vi "main OP500P.vi"() -> ()   [LabVIEW 2020]
uses:
  SubVI/Contactor_Status.ctl
  SubVI/OP500Z8_state_P.ctl
  <userlib>/PCAN Basic/Controls/BaudrateEenum.ctl
  <userlib>/PCAN Basic/Controls/Channel.ctl
  ZEN8 Semi Auto EMC/OP700/SubVI/FGV/FGV_Enum.ctl
  C:/Users/elhajj/OneDrive - FORSEE POWER/Bureau/Support banc de test/Ligne ZENPLUS/Code LabVIEW/CODE/02 SLIM ZEN WS 500/SubVi/FGV.ctl
  13eb9333-f902-445b-951f-98894687dcd3.vi
  af390806-a127-4432-953e-00834710d83e.vi
  5474c4f2-57a2-4d07-9e76-894820534c83.vi
  c213c121-1213-470d-a8c3-6a59dea4dab1.vi
  060584ca-cb65-487f-8f54-703ff4f80a18.vi
  4a804ed1-565a-41e0-a699-ae70de0a1211.vi
  bf7a2284-f80f-49aa-8a3b-6e4a3f45e645.vi
  VG/VG_Barre_Progression_ISO_P.vi
  VG/VG_Ibms.vi
  VG/VG_progressBar_P.vi
  DiagTool/RAMPAGE V1.0/VI/CheminDeBase.vi
  VG/VG_DCIR+OUIouNON_P.vi
  <vilib>/Utility/file.llb/Read Delimited Spreadsheet (string).vi
  VG/VG_Conti.vi
  VG/VG_ISOmin_P.vi
  VG/VG_OCV70min_P.vi
  VG/VG_OCV70max_P.vi
  VG/VG_OCV30max_P.vi
  VG/VG_OCV30min_P.vi
  VG/IS30%_P.vi
  VG/VG_DCIRmax_P.vi
  VG/VG_DCIRmin_P.vi
  <userlib>/PCAN Basic/PCANBasic.lvlib
  <userlib>/Alex_Peak_lib/PEAK_lib_ALEX.lvlib
panel:
  out "Courant BMS (A)":dbl
  out "Consigne ITECH (A)":dbl
  out "Contacteur Status":T1
  out "Boolean":bool
  out "DCIR+ ?":bool
  out "Barre de progression ISO":dbl(slide) scale=0.0..100.0
  out "VISA OUT":T2
  out "IS30% ?":bool
  out "Cluster":T3
  out "progression":dbl(slide) scale=0.0..100.0
  out "errout":errorcluster caption="sortie d'erreur"
  out "STOP":bool
  out "TOP":string
  out "DRAW":picture
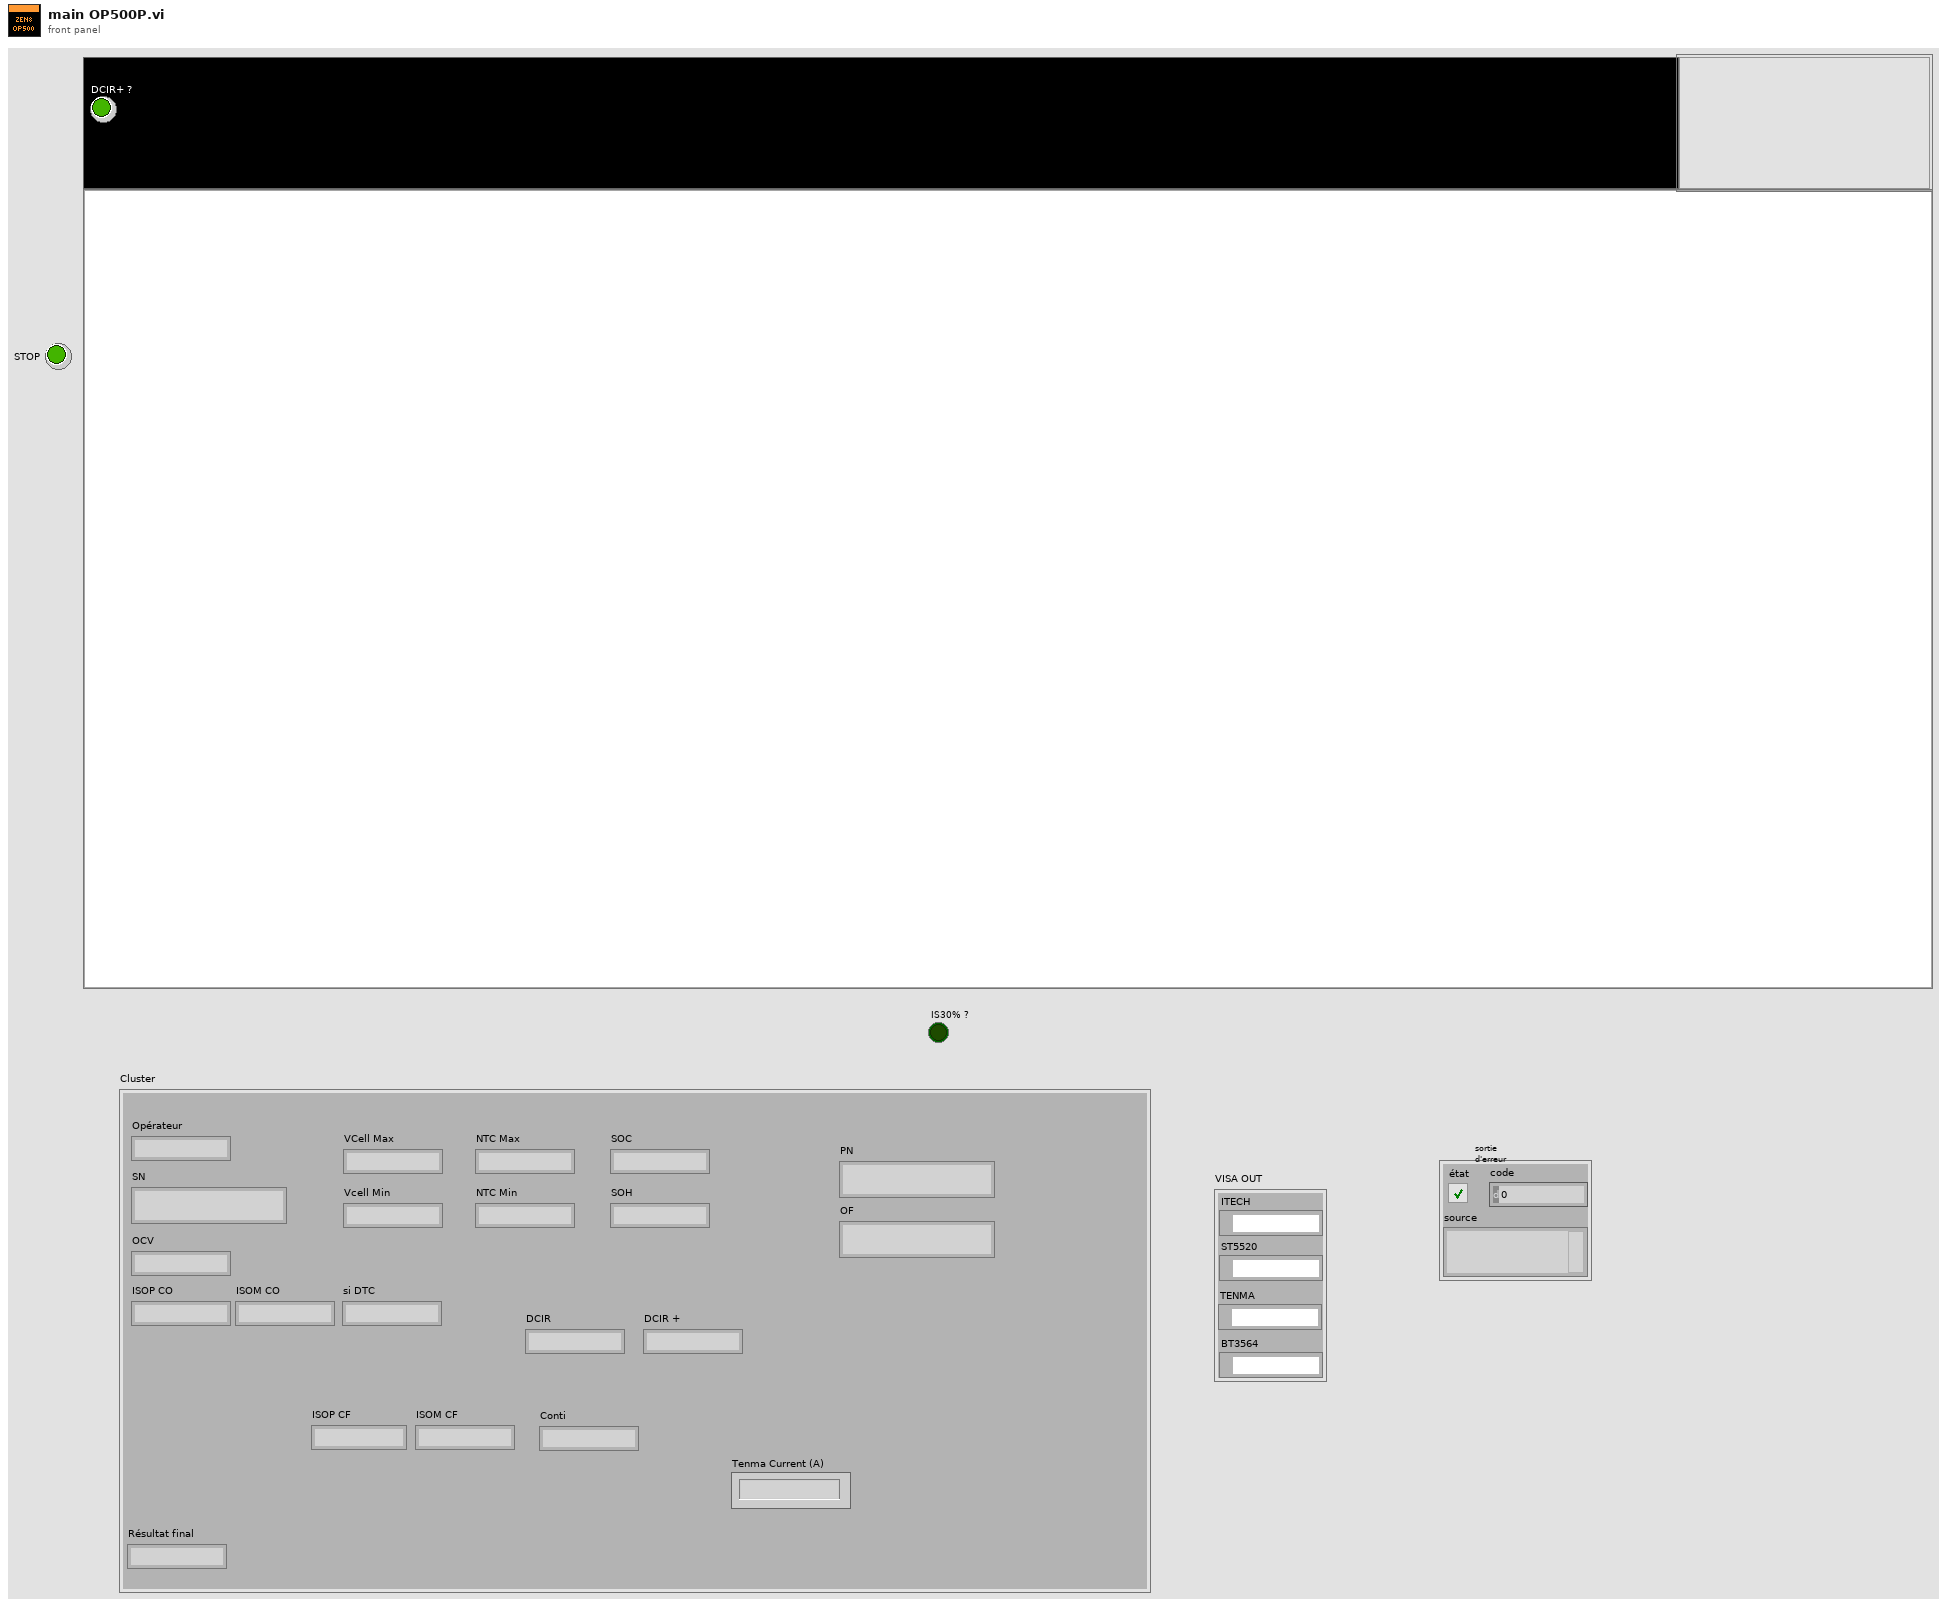
[diagram p1: front panel]
types:
  T1 = typedef "Contactor_Status.ctl" = bool
  T2 = cluster{"ITECH":refnum<visa-resource-name>, "ST5520":refnum<visa-resource-name>, "TENMA":refnum<visa-resource-name>, "BT3564":refnum<visa-resource-name>}
  T3 = cluster{"Opérateur":string, "OCV":string, "ISOP CO":string, "ISOM CO":string, "Résultat final":string, "SN":string, "DCIR":string, "si DTC":string, "Vcell Min":string, "VCell Max":string, "NTC Max":string, "NTC Min":string, "SOC":string, "SOH":string, "PN":string, "OF":string, "DCIR +":string, "Conti":string, "ISOP CF":string, "ISOM CF":string, "Tenma Current (A)":string}
  T4 = typedef "PCANBasic.lvlib/Channel.ctl" = enum16{"PCAN_NONEBUS", "not used1", "not used2", "not used3", "not used4", "not used5", "not used6", "not used7", "not used8", "not used9", "not used10", "not used11", "not used12", "not used13", "not used14", "not used15", "not used16", "not used17", "not used18", "not used19", "not used20", "not used21", "not used22", "not used23", "not used24", "not used25", "not used26", "not used27", "not used28", "not used29", "not used30", "not used31", "not used32", "PCAN_ISABUS1", "PCAN_ISABUS2", "PCAN_ISABUS3", "PCAN_ISABUS4", "PCAN_ISABUS5", "PCAN_ISABUS6", "PCAN_ISABUS7", "PCAN_ISABUS8", "not used41", "not used42", "not used43", "not used44", "not used45", "not used46", "not used47", "not used48", "PCAN_DNGBUS1", "not used50", "not used51", "not used52", "not used53", "not used54", "not used55", "not used56", "not used57", "not used58", "not used59", "not used60", "not used61", "not used62", "not used63", "not used64", "PCAN_PCIBUS1", "PCAN_PCIBUS2", "PCAN_PCIBUS3", "PCAN_PCIBUS4", "PCAN_PCIBUS5", "PCAN_PCIBUS6", "PCAN_PCIBUS7", "PCAN_PCIBUS8", "not used73", "not used74", "not used75", "not used76", "not used77", "not used78", "not used79", "not used80", "PCAN_USBBUS1", "PCAN_USBBUS2", "PCAN_USBBUS3", "PCAN_USBBUS4", "PCAN_USBBUS5", "PCAN_USBBUS6", "PCAN_USBBUS7", "PCAN_USBBUS8", "Not used89", "Not used90", "Not used91", "Not used92", "Not used93", "Not used94", "Not used95", "Not used96", "PCAN_PCCBUS1", "PCAN_PCCBUS2"}
  T5 = typedef "PCANBasic.lvlib/BaudrateEenum.ctl" = enum16{"CAN_Baud_1M", "CAN_Baud_800K", "CAN_BAUD_500K", "CAN_BAUD_250K", "CAN_BAUD_125K", "CAN_BAUD_100K", "CAN_BAUD_95K", "CAN_BAUD_83K", "CAN_BAUD_50K", "CAN_BAUD_47K", "CAN_BAUD_33K", "CAN_BAUD_20K", "CAN_BAUD_10K", "CAN_BAUD_5K", "User Baudrate"}
  T6 = typedef "FGV_Enum.ctl" = enum16{"GET", "SET"}
  T7 = typedef "OP500Z8_state_P.ctl" = enum16{"BuildSys", "Soft", "FinVol", "Null", "Demarrage", "Init", "Scan", "Montage", "Conti", "Iso", "CANCOM", "OCV", "CurrentTest", "GoDCIR", "DataDyn", "Demontage", "Crash", "Next", "DCIR", "EXIT", "LogErr", "DTC"}
  T8 = typedef "FGV.ctl" = enum16{"GET", "SET", "RAZ"}
  T9 = cluster{"OCV":string, "Current":string, "VCell Max":string, "VCell Min":string, "NTC Max":string, "NTC Min":string, "SOC":string, "SOH":string, "DTC":string, "DCIR -":string, "DCIR +":string}
  T10 = cluster{"Opérateur":string, "OCV":string, "ISOP":string, "ISOM":string, "Résultat final":string, "SN":string, "DCIR":string, "si DTC":string, "Vcell Min":string, "VCell Max":string, "NTC Max":string, "NTC Min":string, "SOC":string, "SOH":string, "PN":string, "OF":string, "DCIR+":string, "Conti":string, "ISOP CF":string, "ISOM CF":string, "Tenma Current (A)":string}
  T11 = typedef "imagedata.ctl" = cluster{"image type":i32, "image depth":i32, "image":u8[], "mask":u8[], "colors":u32[], "Rectangle":cluster{"left":i16, "top":i16, "right":i16, "bottom":i16}}
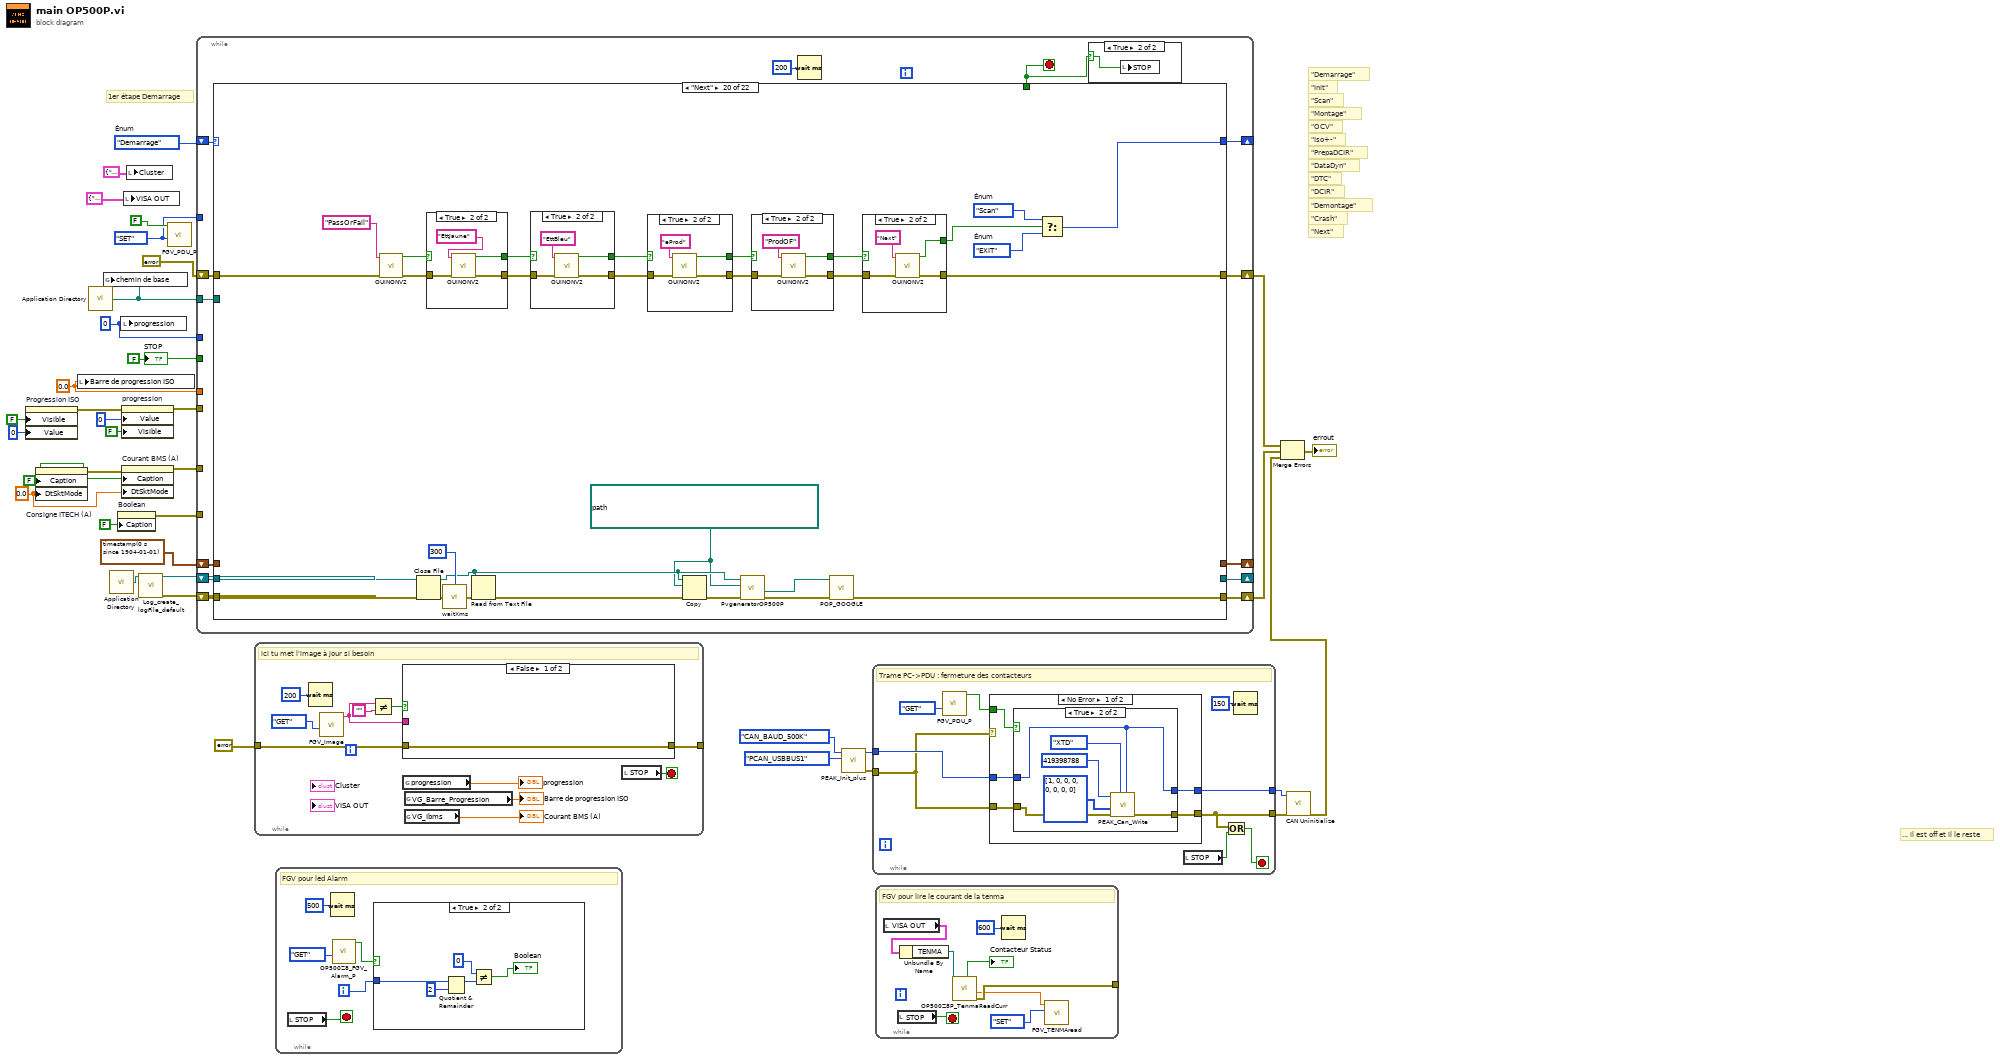
[diagram p0: block diagram]
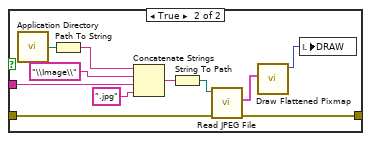
[diagram p5: hidden frame]
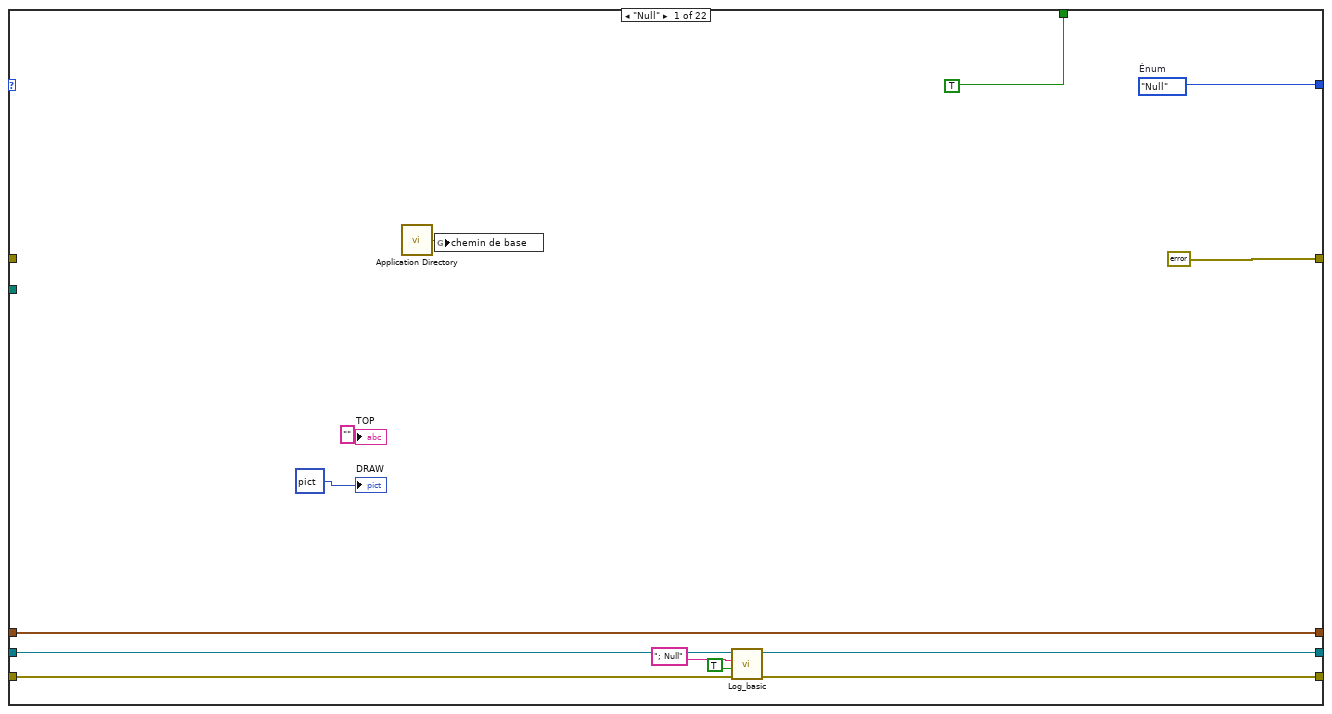
[diagram p7: hidden frame]
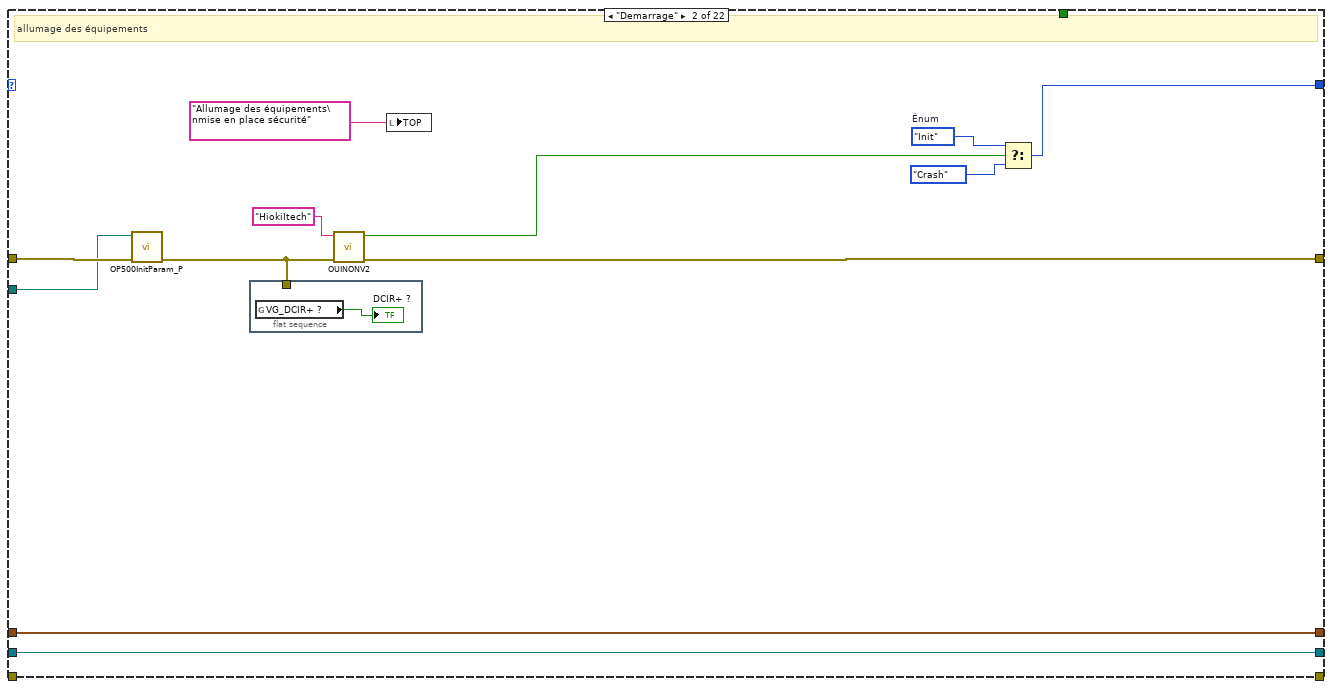
[diagram p8: hidden frame]
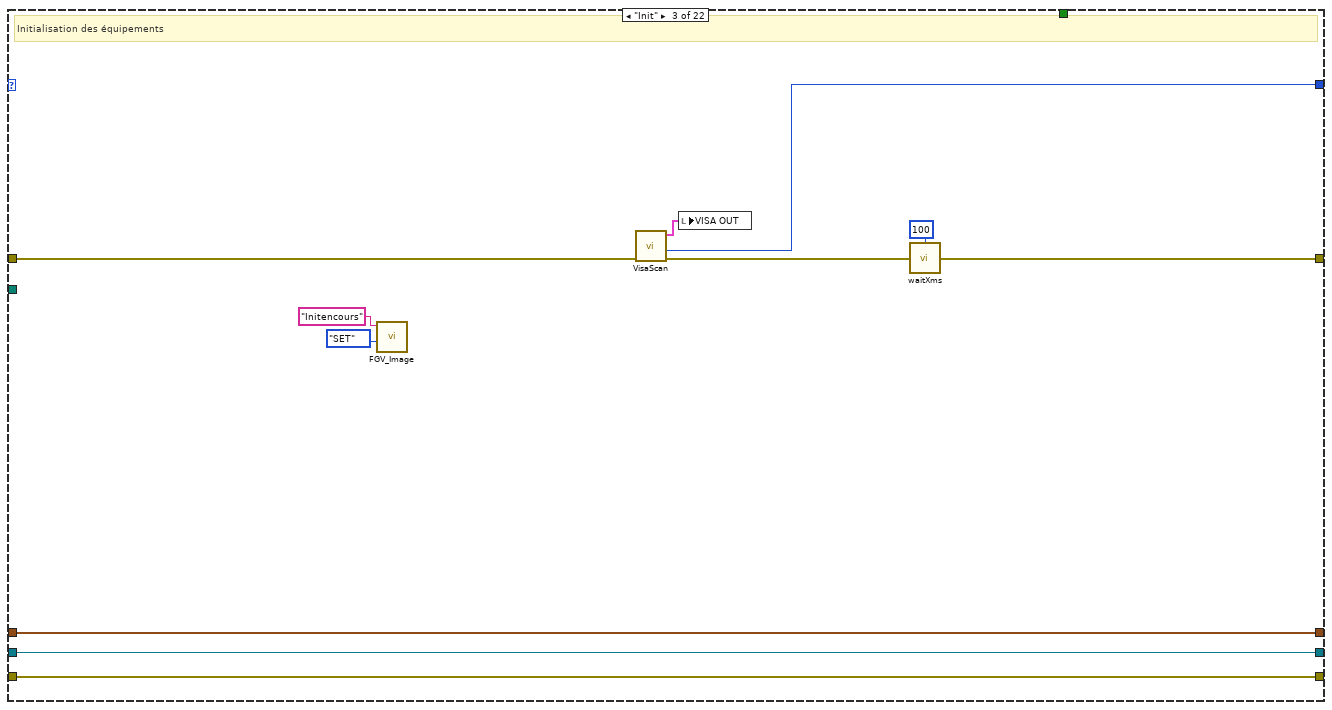
[diagram p9: hidden frame]
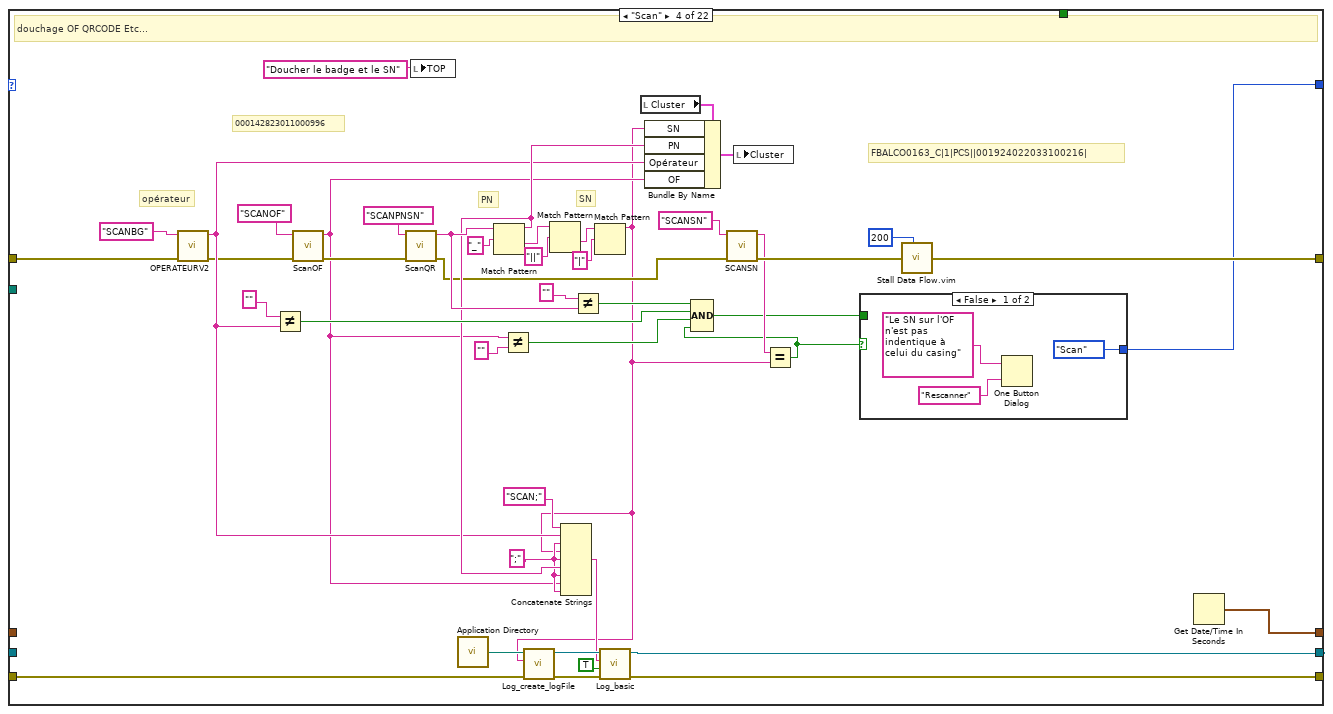
[diagram p10: hidden frame]
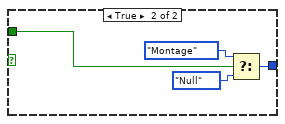
[diagram p11: hidden frame]
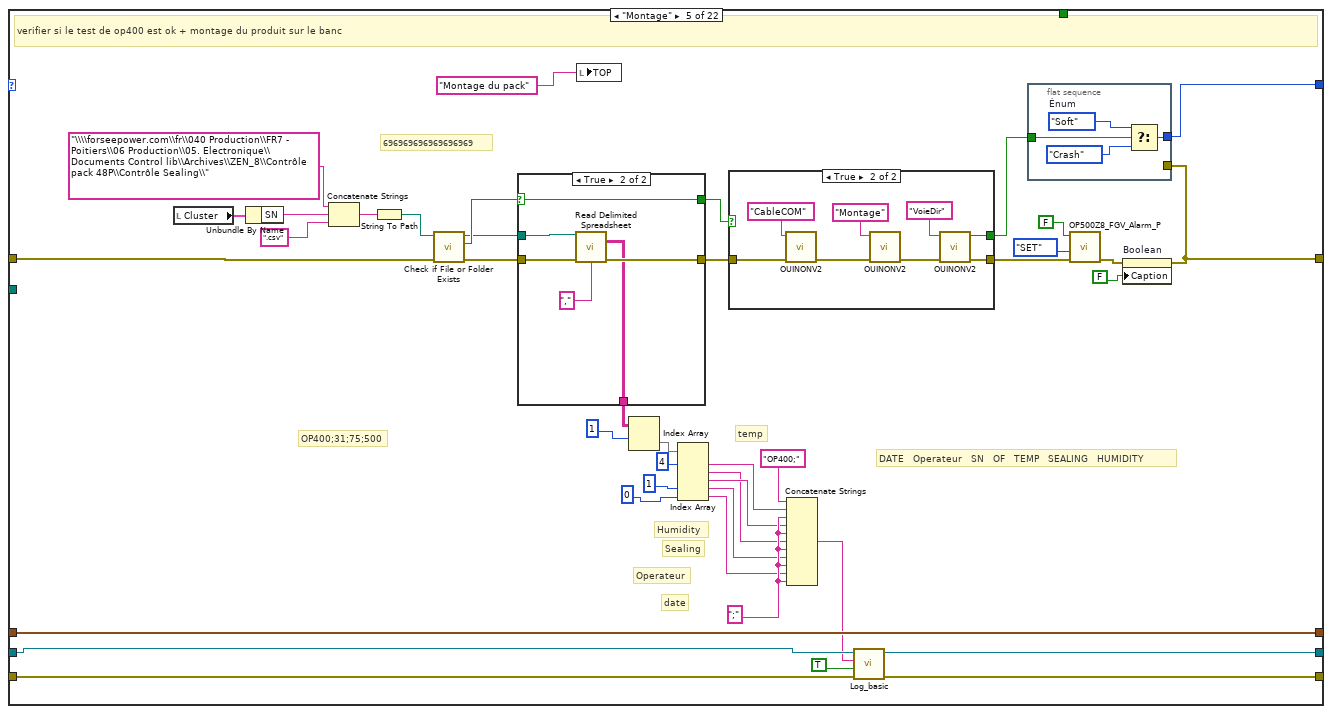
[diagram p12: hidden frame]
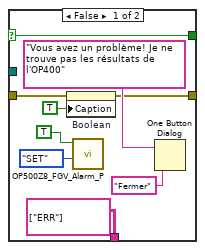
[diagram p14: hidden frame]
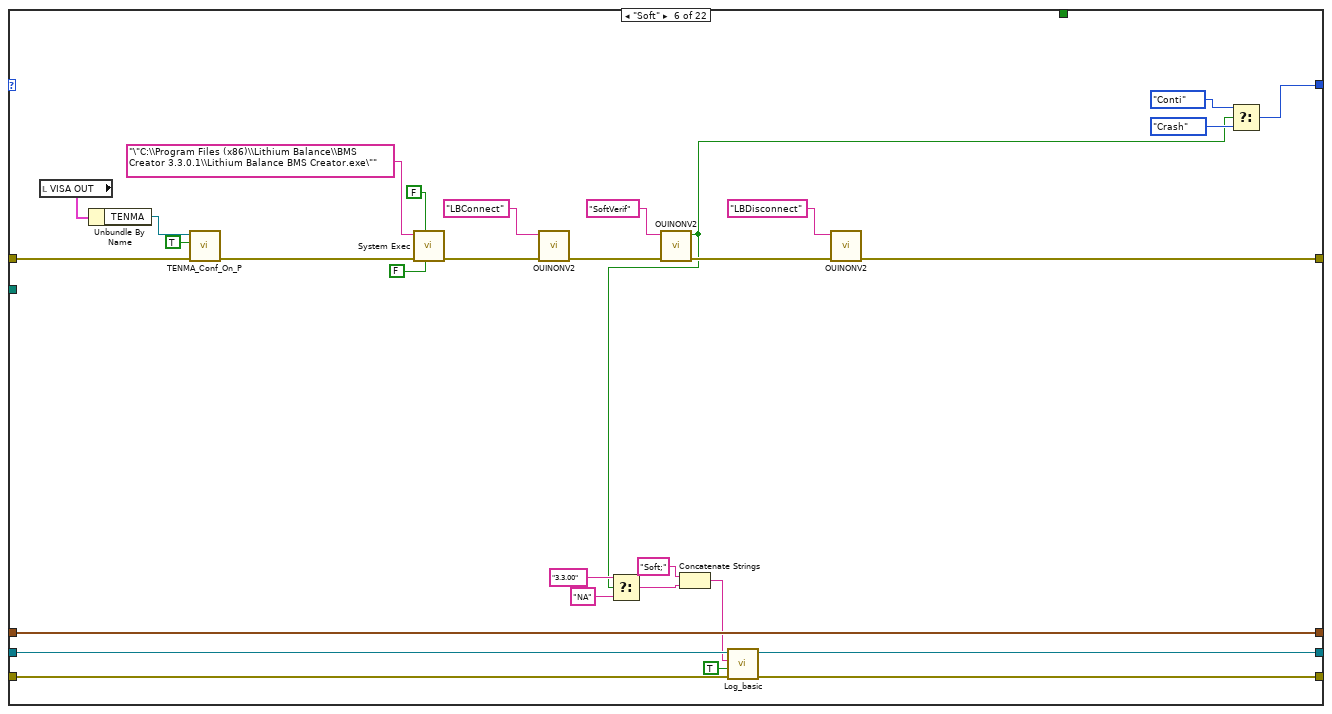
[diagram p15: hidden frame]
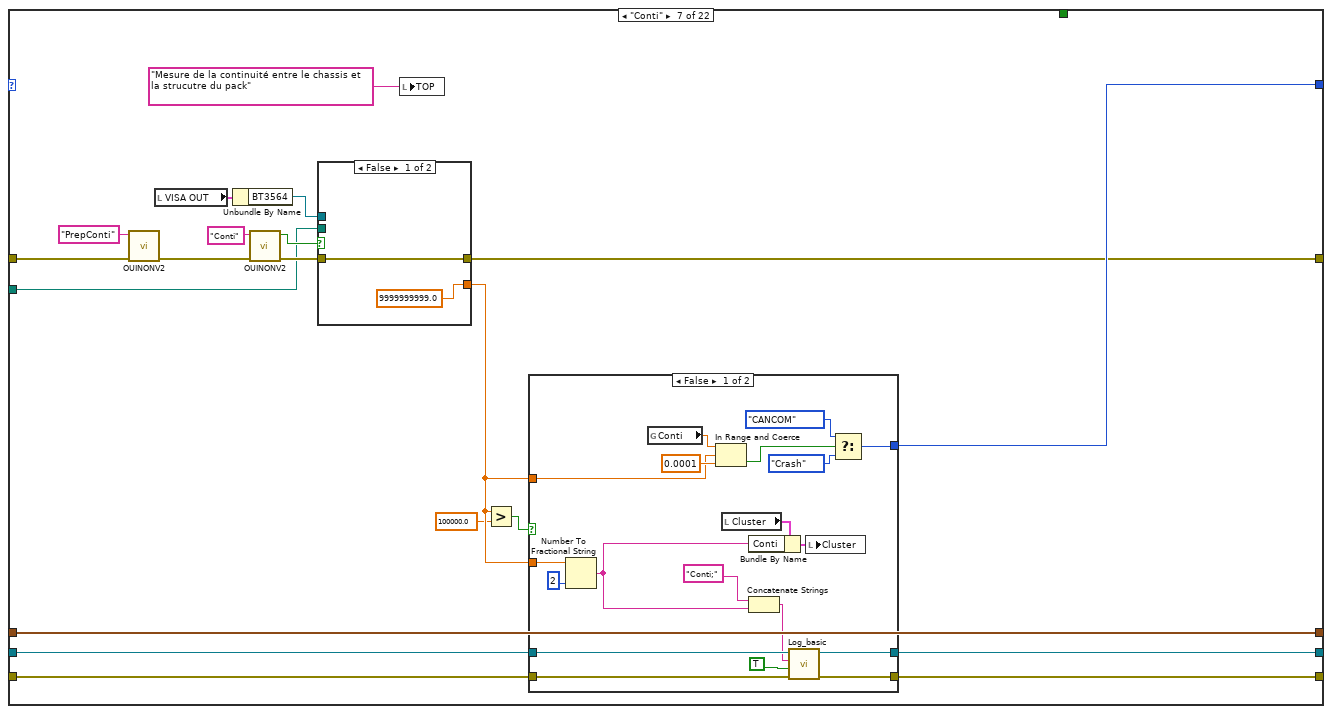
[diagram p16: hidden frame]
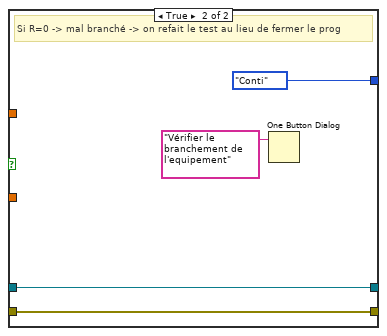
[diagram p17: hidden frame]
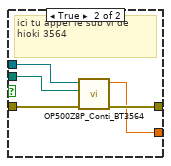
[diagram p18: hidden frame]
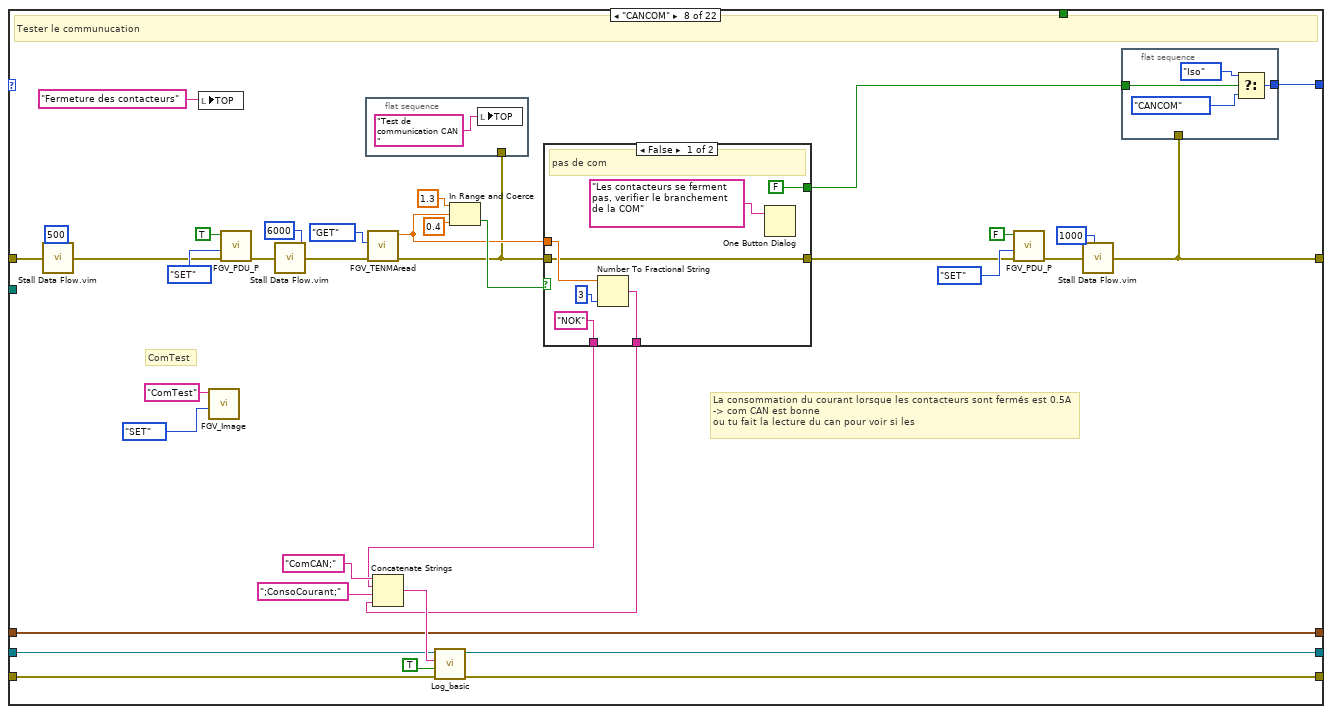
[diagram p19: hidden frame]
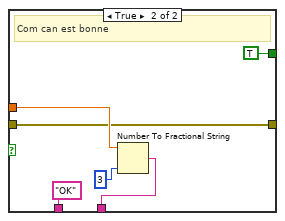
[diagram p20: hidden frame]
diagram:
  w7 = 0.0 ("Consigne ITECH (A)")
  w10 = FALSE ("Caption")
  w16 = FGV_Enum."SET" ("Énum")
  w18 = 0.0 ("Barre de progression ISO")
  w27 = u8 0 ("progression")
  w22 = OP500Z8_state_P."Demarrage"  # Énum
  w33 = FALSE ("STOP")
  # "\"Next\""
  # "\"DCIR\""
  # "\"DTC\""
  # "1er étape Demarrage"
  # "\"Crash\""
  # "\"Demontage\""
  # "\"DataDyn\""
  # "\"Iso+-\""
  # "\"Montage\""
  # "\"Scan\""
  # "\"Init\""
  # "\"Demarrage\""
  # "\"OCV\""
  # "\"PrepaDCIR\""
  # "... il est off et il le reste"
  n1 = property on="Progression ISO" class="Slide (strict)"("Visible"=FALSE, "Value"=u8 0 ("Glissière")) -> (error out=w11:errorcluster)  [unwired: 2 in, 1 out]
  n2 = property on="Consigne ITECH (A)" class="DigNum (strict)"("Caption"=w10, "DtSktMode"=w7) -> (error out=w8:errorcluster)  [unwired: 2 in, 1 out]
  n3 = local write "Barre de progression ISO"(w18) -> ()
  n4 = call <vilib>:"Application Directory.vi"() -> ("Application Directory"=w32:path)
  n5 = global write "CheminDeBase.vi" "chemin de base"(w32) -> ()
  n6 = call <vilib>:"Application Directory.vi"() -> ("Application Directory"=w30:path)
  n7 = property on="Boolean" class="Bool (strict)"("Caption"=FALSE) -> (error out=w13:errorcluster)  [unwired: 2 in, 1 out]
  n8 = local write "progression"(w27) -> ()
  n9 = property on="progression" class="Slide (strict)"(error in=w11, "Value"=u8 0 ("progression"), "Visible"=FALSE) -> (error out=w25:errorcluster)  [unwired: 1 in, 1 out]
  n10 = property on="Courant BMS (A)" class="DigNum (strict)"(error in=w8, "Caption"=w10, "DtSktMode"=w7) -> (error out=w9:errorcluster)  [unwired: 1 in, 1 out]
  n11 = local write "VISA OUT"(T2 {"ITECH"="", "ST5520"="", "TENMA"="", "BT3564"=""} ("VISA OUT")) -> ()
  n12 = local write "Cluster"(T3 {"Opérateur"="", "OCV"="", "ISOP CO"="", "ISOM CO"="", "Résultat final"="", "SN"="", "DCIR"="", "si DTC"="", "Vcell Min"="", "VCell Max"="", "NTC Max"="", "NTC Min"="", "SOC"="", "SOH"="", "PN"="", "OF"="", "DCIR +"="", "Conti"="", "ISOP CF"="", "ISOM CF"="", "Tenma Current (A)"=""} ("Cluster")) -> ()
  n13 = call <userlib>:"Log_create_logFile_default.vi"("appdir"=w30) -> ("errout"=w31:errorcluster, "Fichier à flux d'octets en sortie"=w34:refnum<file>)  [unwired: 9 in]
  n14 = call "FGV_PDU_P.vi"("Énum"=w16, "IN"=FALSE) -> ()  [unwired: 8 in, 2 out]
  n15 = while {
    shift-right: [w49] -> w36
    shift-left: errorcluster {"status"=FALSE, "code"=0, "source"=""} ("error out") -> [w40]
    shift-right: [w45] -> w35
    shift-left: w31 -> [w48]
    shift-right: [w46] -> _
    shift-left: w34 -> [w47]
    tunnel: w32 -> [w43]
    tunnel: w33 -> [_]
    shift-right: [w41] -> _
    shift-left: timestamp(0 s since 1904-01-01) ("seconds since 1Jan1904") -> [w42]
    tunnel: w27 -> [_]
    tunnel: w25 -> [_]
    shift-right: [w38] -> _
    shift-left: w22 -> [w39]
    tunnel: w18 -> [_]
    tunnel: w16 -> [_]
    tunnel: w13 -> [_]
    tunnel: w9 -> [_]
    stop <- w44 stop-if-true
    n16 = case "Structure Condition" shown="\"Next\"" w39 {
      tunnel: w40 -> [_ w69 w83 w133 w170 w214 w244 w292 w350 w463 w524 w607 w727 w750 w776 w796 w837 w854 w862 w898 w951 w957]
      tunnel: [errorcluster {"status"=FALSE, "code"=0, "source"=""} ("errin") w67 w79 w99 w151 w232 w241 w297 w359 w470 w529 w600 w721 w749 w775 w801 w837 w848 w863 w887 w950 w958] -> w49
      tunnel: w48 -> [w60 _ w88 w129 w160 w228 w258 w324 w396 w486 w588 w608 w736 w758 w783 w817 w842 w856 w882 w914 _ _]
      tunnel: w47 -> [w61 w76 w87 _ w158 w227 w260 w323 w395 w488 w590 w609 w734 w757 w788 w819 w844 w857 w883 w915 _ _]
      tunnel: [w58 w76 w87 w131 w141 w226 w256 w317 w394 w484 w586 w609 w733 w756 w789 w820 w845 w857 _ _ _ _] -> w46
      tunnel: [w59 _ w88 w132 w159 w229 w257 w318 w397 w485 w587 w608 w735 w758 w790 w821 w846 w856 w872 w903 _ _] -> w45
      tunnel: [TRUE _ _ _ _ _ _ _ _ _ _ _ _ _ _ _ _ FALSE w884 _ _ _] -> w44
      tunnel: w43 -> [_ w65 _ _ _ _ w249 _ w373 _ _ _ _ _ _ _ _ _ _ _ _ _]
      tunnel: w42 -> [w54 w75 w86 _ w181 w240 w259 w322 w393 w487 w589 w611 w726 _ _ _ _ w853 _ _ _ _]
      tunnel: [w54 w75 w86 w120 w181 w240 w259 w322 w393 w487 w589 w611 w726 _ _ _ _ w853 _ _ _ _] -> w41
      tunnel: [w52 w70 w82 w90 w178 w218 w248 w320 w386 w469 w556 w606 w715 w746 w778 w814 w839 w849 w867 w904 w947 w959] -> w38
      frame "Null" {
        w52 = OP500Z8_state_P."Null"  # Énum
        n17 = call <vilib>:"Application Directory.vi"() -> ("Application Directory"=w64:path)
        n18 = global write "CheminDeBase.vi" "chemin de base"(w64) -> ()
        n19 = call <userlib>:"Log_basic.vi"("errin"=w60, "date?"=TRUE, "chaîne"="; Null", "in"=w61) -> ("sortie d'erreur"=w59:errorcluster, "refnum en sortie"=w58:refnum<file>)  [unwired: 6 in]
        "DRAW" <- picture data[5B] ("DRAW")
        "TOP" <- "" ("TOP")
      }
      frame "Demarrage" {
        w72 = OP500Z8_state_P."Init"  # Énum
        # "allumage des équipements"
        n20 = call "OP500InitParam_P.vi"("errin"=w69, "pathin"=w65) -> ("errout"=w66:errorcluster)  [unwired: 9 in]
        n21 = flat-sequence {
          tunnel: w66 -> [_]
          frame #0 {
            n22 = global read "VG_DCIR+OUIouNON_P.vi" "VG_DCIR+ ?"() -> (→"DCIR+ ?":bool)
          }
        }
        n23 = call <userlib>:"OUINONV2.vi"("errin"=w66, "image"="HiokiItech") -> ("error out"=w67:errorcluster, "Booléen"=w68:bool)  [unwired: 8 in]
        n24 = local write "TOP"("Allumage des équipements\nmise en place sécurité" ("TOP")) -> ()
        n25 = Select ("Sélectionner")(t=w72, s=w68, f=OP500Z8_state_P."Crash" ("cas faux")) -> (s? t:f=w70:T7)
      }
      frame "Init" {
        # "Initialisation des équipements"
        n26 = call "FGV_Image.vi"("Énum"=FGV."SET", "IN"="Initencours") -> ()  [unwired: 9 in, 1 out]
        n27 = call <userlib>:"VisaScan.vi"("errin"=w83) -> ("errout"=w80:errorcluster, "NextStep"=w82:T7, "VISA OUT"=w78:T2)  [unwired: 8 in]
        n28 = local write "VISA OUT"(w78) -> ()
        n29 = call <userlib>:"waitXms.vi"("attente (ms)"=u32 100, "errin"=w80) -> ("errout"=w79:errorcluster)  [unwired: 13 in]
      }
      frame "Scan" {
        w103 = ";" ("chaîne")
        # "SN"
        # "PN"
        # "FBALCO0163_C|1|PCS||001924022033100216|"
        # "000142823011000996"
        # "opérateur"
        # "douchage OF QRCODE Etc..."
        n30 = call "OPERATEURV2.vi"("errin"=w133, "IN"="SCANBG") -> ("error out"=w102:errorcluster, "Dataout"=w107:string)  [unwired: 8 in]
        n31 = Not Equal?(x="", y=w107) -> (x != y?=w121:bool)
        n32 = call <userlib>:"ScanOF.vi"("errin"=w102, "image"="SCANOF") -> ("error out"=w101:errorcluster, "OF"=w97:string)  [unwired: 8 in]
        n33 = call <userlib>:"ScanQR.vi"("errin"=w101, "image"="SCANPNSN") -> ("error out"=w96:errorcluster, "OF"=w114:string)  [unwired: 7 in, 1 out]
        n34 = local write "TOP"("Doucher le badge et le SN" ("TOP")) -> ()
        n35 = call <vilib>:"Application Directory.vi"() -> ("Application Directory"=w130:path)
        n36 = Match Pattern(string=w114, regular expression="_" ("expression régulière")) -> (before substring=w108:string, after substring=w112:string)  [unwired: 1 in, 2 out]
        n37 = Not Equal?(x=w97, y="") -> (x != y?=w104:bool)
        n38 = Match Pattern(string=w112, regular expression="||" ("expression régulière")) -> (after substring=w110:string)  [unwired: 1 in, 3 out]
        n39 = Not Equal?(x="", y=w114) -> (x != y?=w122:bool)
        n40 = Match Pattern(string=w110, regular expression="|" ("expression régulière")) -> (before substring=w92:string)  [unwired: 1 in, 3 out]
        n41 = call <userlib>:"Log_create_logFile.vi"("errin"=w129, "toute l'expression"=w92, "Application Directory"=w130) -> ("sortie d'erreur"=w127:errorcluster, "Fichier à flux d'octets en sortie"=w128:refnum<file>)  [unwired: 7 in]
        n42 = Concatenate Strings("SCAN;" ("chaîne"), w107, w103, w92, w103, w108, w103, w97, w103) -> (w125:string)
        n43 = call <userlib>:"Log_basic.vi"("errin"=w127, "date?"=TRUE, "chaîne"=w125, "in"=w128) -> ("sortie d'erreur"=w132:errorcluster, "refnum en sortie"=w131:refnum<file>)  [unwired: 6 in]
        n44 = local read "Cluster"() -> (w116:T3)
        n45 = Bundle By Name(cluster=w116, "SN"=w92, "PN"=w108, "Opérateur"=w107, "OF"=w97) -> (w115:T3)
        n46 = call <userlib>:"SCANSN.vi"("errin"=w96, "image"="SCANSN") -> ("error out"=w95:errorcluster, "SN"=w93:string)  [unwired: 8 in]
        n47 = local write "Cluster"(w115) -> ()
        n48 = Equal?(x=w93, y=w92) -> (x = y?=w91:bool)
        n49 = Compound Arithmetic op=AND ("Opérateur arithmétique")(w122, w121, w104, w91) -> (w89:bool)
        n50 = case shown="False" w91 {
          tunnel: [OP500Z8_state_P."Scan" ("cas faux") w138] -> w90
          tunnel: w89 -> [_ w137]
          frame False {
            n51 = One Button Dialog(message="Le SN sur l'OF n'est pas indentique à celui du casing", button name ("OK")="Rescanner" ("nom du bouton (\"OK\")")) -> ()  [unwired: 1 out]
          }
          frame True {
            n52 = Select ("Sélectionner")(t=OP500Z8_state_P."Montage" ("Énum"), s=w137, f=OP500Z8_state_P."Null" ("cas faux")) -> (s? t:f=w138:T7)
          }
        }
        n53 = call "Stall Data Flow.vim"("value in"=w95, "milliseconds to wait"=u32 200) -> ("value out"=w99:errorcluster)  [unwired: 1 out]
        n54 = Get Date/Time In Seconds() -> (seconds since 1Jan1904=w120:timestamp)
      }
      frame "Montage" {
        w150 = ";" ("string")
        # "date"
        # "OP400;31;75;500"
        # "Sealing"
        # "Operateur"
        # "Humidity"
        # "temp"
        # "DATE   Operateur   SN   OF   TEMP   SEALING   HUMIDITY"
        # "696969696969696969"
        # "verifier si le test de op400 est ok + montage du produit sur le banc"
        n55 = local read "Cluster"() -> (w177:T3)
        n56 = Unbundle By Name(w177) -> ("SN"=w176:string)
        n57 = Concatenate Strings("\\\\forseepower.com\\fr\\040 Production\\FR7 - Poitiers\\06 Production\\05. Electronique\\Documents Control lib\\Archives\\ZEN_8\\Contrôle pack 48P\\Contrôle Sealing\\" ("string"), w176, ".csv" ("string")) -> (w173:string)
        n58 = String To Path(string=w173) -> (path=w171:path)
        n59 = call <vilib>:"Check if File or Folder Exists.vi"("error in (no error)"=w170, "path"=w171) -> ("error out"=w169:errorcluster, "file or folder exists?"=w168:bool, "dup path"=w166:path)  [unwired: 7 in]
        n60 = case shown="True" w168 {
          selector: w168 -> [w204 w207]
          tunnel: [w199 w209] -> w172
          tunnel: w169 -> [w200 w208]
          tunnel: [w204 w207] -> w167
          tunnel: w166 -> [_ w206]
          tunnel: [string[][] [["ERR"]] ("all rows") w205] -> w153
          frame False {
            n61 = property on="Boolean" class="Bool (strict)"(error in=w200, "Caption"=TRUE) -> (error out=w199:errorcluster)  [unwired: 1 in, 1 out]
            n62 = call "OP500Z8_FGV_Alarm_P.vi"("Énum"=FGV_Enum."SET", "IN"=TRUE) -> ()  [unwired: 8 in, 2 out]
            n63 = One Button Dialog(message="Vous avez un problème! Je ne trouve pas les résultats de l'OP400", button name ("OK")="Fermer") -> ()  [unwired: 1 out]
          }
          frame True {
            n64 = call-poly <vilib>:"Read Delimited Spreadsheet.vi"("file path (dialog if empty)"=w206, "error in (no error)"=w208, "delimiter (\\t)"="," ("delimiter (\\t)")) -> ("all rows"=w205:string[][], "error out"=w209:errorcluster)  [unwired: 7 in, 4 out]
          }
        }
        n65 = local write "TOP"("Montage du pack" ("TOP")) -> ()
        n66 = Index Array(array=w153, index (row)=1) -> (element=w152:string[])  [unwired: 1 in]
        n67 = Index Array(array=w152, index #1=4 ("index"), index #4=1 ("index"), index #5=0 ("index")) -> (element #1=w148:string, element #2=w145:string, element #3=w146:string, element #4=w144:string, element #5=w142:string)  [unwired: 2 in]
        n68 = case shown="True" w167 {
          selector: w167 -> [w186 _]
          tunnel: [w187 w189] -> w165
          tunnel: [w186 w188] -> w180
          tunnel: w172 -> [w187 w191]
          frame False {
          }
          frame True {
            n69 = call <userlib>:"OUINONV2.vi"("errin"=w191, "image"="CableCOM") -> ("error out"=w190:errorcluster)  [unwired: 8 in, 1 out]
            n70 = call <userlib>:"OUINONV2.vi"("errin"=w190, "image"="Montage" ("IN")) -> ("error out"=w193:errorcluster)  [unwired: 8 in, 1 out]
            n71 = call <userlib>:"OUINONV2.vi"("errin"=w193, "image"="VoieDir") -> ("error out"=w189:errorcluster, "Booléen"=w188:bool)  [unwired: 8 in]
          }
        }
        n72 = Concatenate Strings("OP400;" ("string"), w148, w150, w146, w150, w145, w150, w144, w150, w142, w150) -> (w156:string)
        n73 = call <userlib>:"Log_basic.vi"("errin"=w160, "date?"=TRUE, "chaîne"=w156, "in"=w158) -> ("sortie d'erreur"=w159:errorcluster, "refnum en sortie"=w141:refnum<file>)  [unwired: 6 in]
        n74 = flat-sequence {
          tunnel: w180 -> [w185]
          tunnel: [w182] -> w178
          tunnel: w151 -> [_]
          frame #0 {
            w184 = OP500Z8_state_P."Soft"  # Énum
            n75 = Select ("Sélectionner")(t=w184, s=w185, f=OP500Z8_state_P."Crash" ("cas faux")) -> (s? t:f=w182:T7)
          }
        }
        n76 = call "OP500Z8_FGV_Alarm_P.vi"("errin"=w165, "Énum"=FGV_Enum."SET", "IN"=FALSE) -> ("errout"=w161:errorcluster)  [unwired: 7 in, 1 out]
        n77 = property on="Boolean" class="Bool (strict)"(error in=w161, "Caption"=FALSE) -> (error out=w151:errorcluster)  [unwired: 1 in, 1 out]
      }
      frame "Soft" {
        n78 = local read "VISA OUT"() -> (w213:T2)
        n79 = Unbundle By Name(w213) -> ("TENMA"=w212:refnum<visa-resource-name>)
        n80 = call "TENMA_Conf_On_P.vi"("errin"=w214, "Tenma On?"=TRUE, "Visa in tenma"=w212) -> ("sortie d'erreur"=w215:errorcluster)  [unwired: 7 in, 1 out]
        n81 = call <vilib>:"System Exec.vi"("run minimized? (F)"=FALSE, "wait until completion? (T)"=FALSE, "error in (no error)"=w215, "command line"="\"C:\\Program Files (x86)\\Lithium Balance\\BMS Creator 3.3.0.1\\Lithium Balance BMS Creator.exe\"") -> ("error out"=w238:errorcluster)  [unwired: 4 in, 3 out]
        n82 = call <userlib>:"OUINONV2.vi"("errin"=w238, "image"="LBConnect" ("command line")) -> ("error out"=w236:errorcluster)  [unwired: 8 in, 1 out]
        n83 = call <userlib>:"OUINONV2.vi"("errin"=w236, "image"="SoftVerif" ("command line")) -> ("error out"=w231:errorcluster, "Booléen"=w216:bool)  [unwired: 8 in]
        n84 = Select(t="3.3.00" ("string"), s=w216, f="NA") -> (s? t:f=w220:string)
        n85 = Concatenate Strings("Soft;" ("string"), w220) -> (w224:string)
        n86 = call <userlib>:"Log_basic.vi"("errin"=w228, "date?"=TRUE, "chaîne"=w224, "in"=w227) -> ("sortie d'erreur"=w229:errorcluster, "refnum en sortie"=w226:refnum<file>)  [unwired: 6 in]
        n87 = call <userlib>:"OUINONV2.vi"("errin"=w231, "image"="LBDisconnect") -> ("error out"=w232:errorcluster)  [unwired: 8 in, 1 out]
        n88 = Select(t=OP500Z8_state_P."Conti" ("Énum"), s=w216, f=OP500Z8_state_P."Crash") -> (s? t:f=w218:T7)
      }
      frame "Conti" {
        n89 = call <userlib>:"OUINONV2.vi"("errin"=w244, "image"="PrepConti") -> ("error out"=w243:errorcluster)  [unwired: 8 in, 1 out]
        n90 = local read "VISA OUT"() -> (w251:T2)
        n91 = Unbundle By Name(w251) -> ("BT3564"=w250:refnum<visa-resource-name>)
        n92 = call <userlib>:"OUINONV2.vi"("errin"=w243, "image"="Conti" ("IN")) -> ("error out"=w254:errorcluster, "Booléen"=w252:bool)  [unwired: 8 in]
        n93 = case shown="False" w252 {
          tunnel: [w285 w289] -> w241
          tunnel: [9999999999.0 ("Tension Bat+ Bat-") w286] -> w247
          tunnel: w254 -> [w285 w290]
          tunnel: w250 -> [_ w288]
          tunnel: w249 -> [_ w287]
          frame False {
          }
          frame True {
            # "ici tu appel le sub vi de hioki 3564"
            n94 = call "OP500Z8P_Conti_BT3564.vi"("errin"=w290, "chemin de base"=w287, "VISAin"=w288) -> ("errout"=w289:errorcluster, "R mOhm"=w286:dbl)  [unwired: 7 in]
          }
        }
        n95 = local write "TOP"("Mesure de la continuité entre le chassis et la strucutre du pack" ("TOP")) -> ()
        n96 = Greater?(x=w247, y=100000.0) -> (0:w245:bool)
        n97 = case shown="False" w245 {
          tunnel: w260 -> [w279 w282]
          tunnel: w258 -> [w278 w283]
          tunnel: [w277 w283] -> w257
          tunnel: [w276 w282] -> w256
          tunnel: w247 -> [w268 _]
          tunnel: [w262 OP500Z8_state_P."Conti" ("f")] -> w248
          tunnel: w247 -> [w261 _]
          frame False {
            n98 = Number To Fractional String(number=w268, precision (6)=i16 2 ("précision (6)")) -> (F-format string=w273:string)  [unwired: 2 in]
            n99 = global read "VG_Conti.vi" "Conti"() -> (w267:dbl)
            n100 = In Range and Coerce(upper limit=w267, x=w261, lower limit=0.0001) -> (In Range?=w266:bool)  [unwired: 1 out]
            n101 = local read "Cluster"() -> (w275:T3)
            n102 = Bundle By Name(cluster=w275, "Conti"=w273) -> (w274:T3)
            n103 = Concatenate Strings("Conti;" ("chaîne"), w273) -> (w271:string)
            n104 = call <userlib>:"Log_basic.vi"("errin"=w278, "date?"=TRUE, "chaîne"=w271, "in"=w279) -> ("sortie d'erreur"=w277:errorcluster, "refnum en sortie"=w276:refnum<file>)  [unwired: 6 in]
            n105 = local write "Cluster"(w274) -> ()
            n106 = Select(t=OP500Z8_state_P."CANCOM" ("Cas OK"), s=w266, f=OP500Z8_state_P."Crash") -> (s? t:f=w262:T7)
          }
          frame True {
            # "Si R=0 -> mal branché -> on refait le test au lieu de fermer le prog"
            n107 = One Button Dialog(message="Vérifier le branchement de l'equipement") -> ()  [unwired: 1 in, 1 out]
          }
        }
      }
      frame "CANCOM" {
        # "ComTest"
        # "La consommation du courant lorsque les contacteurs sont fermés est 0.5A -> com CAN est bonne\nou tu fait la lecture du can pour voir si les"
        # "Tester le communucation"
        n108 = call "Stall Data Flow.vim"("value in"=w292, "milliseconds to wait"=u32 500) -> ("value out"=w293:errorcluster)  [unwired: 1 out]
        n109 = local write "TOP"("Fermeture des contacteurs" ("TOP")) -> ()
        n110 = call "FGV_Image.vi"("Énum"=FGV."SET", "IN"="ComTest") -> ()  [unwired: 9 in, 1 out]
        n111 = call "FGV_PDU_P.vi"("errin"=w293, "Énum"=FGV_Enum."SET", "IN"=TRUE) -> ("errout"=w304:errorcluster)  [unwired: 7 in, 1 out]
        n112 = call "Stall Data Flow.vim"("value in"=w304, "milliseconds to wait"=u32 6000) -> ("value out"=w303:errorcluster)  [unwired: 1 out]
        n113 = flat-sequence {
          tunnel: w294 -> [_]
          frame #0 {
            n114 = local write "TOP"("Test de communication CAN " ("TOP")) -> ()
          }
        }
        n115 = call "FGV_TENMAread.vi"("errin"=w303, "Énum"=FGV_Enum."GET") -> ("errout"=w294:errorcluster, "Numeric output"=w311:dbl)  [unwired: 8 in]
        n116 = In Range and Coerce(upper limit=1.3, x=w311, lower limit=0.4) -> (In Range?=w313:bool)  [unwired: 1 out]
        n117 = case shown="False" w313 {
          tunnel: w294 -> [w333 w339]
          tunnel: ["NOK" ("TOP") "OK" ("TOP")] -> w312
          tunnel: w311 -> [w336 w343]
          tunnel: [w335 w341] -> w309
          tunnel: [FALSE TRUE] -> w308
          tunnel: [w333 w339] -> w291
          frame False {
            # "pas de com"
            n118 = Number To Fractional String(number=w336, precision (6)=i16 3) -> (F-format string=w335:string)  [unwired: 2 in]
            n119 = One Button Dialog(message="Les contacteurs se ferment pas, verifier le branchement de la COM") -> ()  [unwired: 1 in, 1 out]
          }
          frame True {
            # "Com can est bonne"
            n120 = Number To Fractional String(number=w343, precision (6)=i16 3) -> (F-format string=w341:string)  [unwired: 2 in]
          }
        }
        n121 = Concatenate Strings("ComCAN;" ("string"), w312, ";ConsoCourant;" ("string"), w309) -> (w326:string)
        n122 = call <userlib>:"Log_basic.vi"("errin"=w324, "date?"=TRUE, "chaîne"=w326, "in"=w323) -> ("sortie d'erreur"=w318:errorcluster, "refnum en sortie"=w317:refnum<file>)  [unwired: 6 in]
        n123 = call "FGV_PDU_P.vi"("errin"=w291, "Énum"=FGV_Enum."SET", "IN"=FALSE) -> ("errout"=w299:errorcluster)  [unwired: 7 in, 1 out]
        n124 = call "Stall Data Flow.vim"("value in"=w299, "milliseconds to wait"=u32 1000) -> ("value out"=w297:errorcluster)  [unwired: 1 out]
        n125 = flat-sequence {
          tunnel: [w330] -> w320
          tunnel: w308 -> [w328]
          tunnel: w297 -> [_]
          frame #0 {
            n126 = Select ("Sélectionner")(t=OP500Z8_state_P."Iso" ("cas vrai"), s=w328, f=OP500Z8_state_P."CANCOM" ("Énum")) -> (s? t:f=w330:T7)
          }
        }
      }
      frame "Iso" {
        # "test d'isolement Bat+ et Bat-"
        n127 = call <userlib>:"OUINONV2.vi"("errin"=w350, "image"="ISOSTART") -> ("error out"=w351:errorcluster)  [unwired: 8 in, 1 out]
        n128 = call <userlib>:"OUINONV2.vi"("errin"=w351, "image"="MultiEPI") -> ("error out"=w356:errorcluster, "Booléen"=w357:bool)  [unwired: 8 in]
        n129 = local read "VISA OUT"() -> (w383:T2)
        n130 = local write "TOP"("Test d'isolement BAT+ Contacteurs ouverts" ("TOP")) -> ()
        n131 = case shown="True" w357 {
          selector: w357 -> [w455 _]
          tunnel: [w455 w459] -> w388
          tunnel: [w456 w458] -> w354
          tunnel: w356 -> [w456 w457]
          frame False {
          }
          frame True {
            n132 = call <userlib>:"OUINONV2.vi"("errin"=w457, "image"="ISOPCO" ("IN")) -> ("error out"=w458:errorcluster, "Booléen"=w459:bool)  [unwired: 8 in]
          }
        }
        n133 = global read "VG_ISOmin_P.vi" "ISOP CO"() -> (w380:dbl)
        n134 = Unbundle By Name(w383) -> ("ST5520"=w370:refnum<visa-resource-name>)
        n135 = flat-sequence {
          tunnel: w354 -> [_]
          frame #0 {
            n136 = local write "TOP"("Test d'isolement BAT-  Contacteurs ouverts" ("TOP")) -> ()
          }
        }
        n137 = control-ref of="BP ISO"() -> (w352:refnum<vi>)
        n138 = call "OP500Z8P_ISOmicro.vi"("reference"=w352, "critere Iso"=w380, "errin"=w354, "Booléen"=w388, "Application Directory"=w373, "VISA Refnum in"=w370) -> ("error out"=w353:errorcluster, "Ok ?"=w379:bool, "String"=w382:string)  [unwired: 3 in]
        n139 = global read "VG_ISOmin_P.vi" "ISOM CO"() -> (w374:dbl)
        n140 = case shown="True" w379 {
          selector: w379 -> [w443 _]
          tunnel: [w441 w451] -> w345
          tunnel: w353 -> [w441 w453]
          tunnel: [w443 w450] -> w378
          tunnel: [w442 w446] -> w377
          tunnel: w374 -> [_ w449]
          tunnel: w370 -> [_ w448]
          tunnel: w373 -> [_ w447]
          tunnel: [w442 w446] -> w368
          tunnel: w352 -> [_ w444]
          frame False {
            w442 = "ISOF" ("String")
          }
          frame True {
            n141 = call <userlib>:"OUINONV2.vi"("errin"=w453, "image"="ISOMCO" ("IN")) -> ("error out"=w445:errorcluster, "Booléen"=w452:bool)  [unwired: 8 in]
            n142 = call "OP500Z8P_ISOmicro.vi"("reference"=w444, "critere Iso"=w449, "errin"=w445, "Booléen"=w452, "Application Directory"=w447, "VISA Refnum in"=w448) -> ("error out"=w451:errorcluster, "Ok ?"=w450:bool, "String"=w446:string)  [unwired: 3 in]
          }
        }
        n143 = flat-sequence {
          tunnel: w348 -> [_]
          frame #0 {
            n144 = local write "TOP"("Test d'isolement BAT+ Contacteurs fermés" ("TOP")) -> ()
          }
        }
        n145 = call "FGV_PDU_P.vi"("errin"=w345, "Énum"=FGV_Enum."SET", "IN"=TRUE) -> ("errout"=w347:errorcluster)  [unwired: 7 in, 1 out]
        n146 = call "Stall Data Flow.vim"("value in"=w347, "milliseconds to wait"=u32 6000) -> ("value out"=w348:errorcluster)  [unwired: 1 out]
        n147 = global read "VG_ISOmin_P.vi" "ISOP CF"() -> (w371:dbl)
        n148 = case shown="True" w378 {
          selector: w378 -> [w429 _]
          tunnel: [w427 w437] -> w358
          tunnel: w348 -> [w427 w439]
          tunnel: [w428 w432] -> w376
          tunnel: [w429 w436] -> w375
          tunnel: w370 -> [_ w435]
          tunnel: w373 -> [_ w434]
          tunnel: w371 -> [_ w433]
          tunnel: [w428 w432] -> w367
          tunnel: w352 -> [_ w430]
          frame False {
            w428 = "ISOF" ("String")
          }
          frame True {
            n149 = call <userlib>:"OUINONV2.vi"("errin"=w439, "image"="ISOPCF" ("IN")) -> ("error out"=w431:errorcluster, "Booléen"=w438:bool)  [unwired: 8 in]
            n150 = call "OP500Z8P_ISOmicro.vi"("reference"=w430, "critere Iso"=w433, "errin"=w431, "Booléen"=w438, "Application Directory"=w434, "VISA Refnum in"=w435) -> ("error out"=w437:errorcluster, "Ok ?"=w436:bool, "String"=w432:string)  [unwired: 3 in]
          }
        }
        n151 = flat-sequence {
          tunnel: w358 -> [_]
          frame #0 {
            n152 = local write "TOP"("Test d'isolement BAT- Contacteurs fermés" ("TOP")) -> ()
          }
        }
        n153 = global read "VG_ISOmin_P.vi" "ISOM CF"() -> (w372:dbl)
        n154 = case shown="True" w375 {
          selector: w375 -> [w415 _]
          tunnel: [w413 w423] -> w363
          tunnel: w358 -> [w413 w425]
          tunnel: [w414 w418] -> w364
          tunnel: w373 -> [_ w422]
          tunnel: [w415 w421] -> w369
          tunnel: w372 -> [_ w420]
          tunnel: w370 -> [_ w419]
          tunnel: [w414 w418] -> w365
          tunnel: w352 -> [_ w416]
          frame False {
            w414 = "ISOF" ("String")
          }
          frame True {
            n155 = call <userlib>:"OUINONV2.vi"("errin"=w425, "image"="ISOMCF" ("IN")) -> ("error out"=w417:errorcluster, "Booléen"=w424:bool)  [unwired: 8 in]
            n156 = call "OP500Z8P_ISOmicro.vi"("reference"=w416, "critere Iso"=w420, "errin"=w417, "Booléen"=w424, "Application Directory"=w422, "VISA Refnum in"=w419) -> ("error out"=w423:errorcluster, "Ok ?"=w421:bool, "String"=w418:string)  [unwired: 3 in]
          }
        }
        n157 = local read "Cluster"() -> (w392:T3)
        n158 = Bundle By Name(cluster=w392, "ISOP CO"=w382, "ISOM CO"=w377, "ISOP CF"=w376, "ISOM CF"=w364) -> (w391:T3)
        n159 = local write "Cluster"(w391) -> ()
        n160 = Concatenate Strings("ISO;" ("string"), "ISO+CO;" ("chaîne"), w382, ";ISO-CO;" ("chaîne"), w368, ";ISO+CF;" ("chaîne"), w367, ";ISO-CF;" ("chaîne"), w365) -> (w401:string)
        n161 = case shown="True" w369 {
          selector: w369 -> [w406 _]
          tunnel: [w405 w412] -> w359
          tunnel: [w406 w411] -> w390
          tunnel: w363 -> [w405 w408]
          frame False {
          }
          frame True {
            n162 = call <userlib>:"OUINONV2.vi"("errin"=w408, "image"="EPIOFF") -> ("error out"=w407:errorcluster)  [unwired: 8 in, 1 out]
            n163 = call <userlib>:"OUINONV2.vi"("errin"=w407, "image"="ISOEND") -> ("error out"=w412:errorcluster, "Booléen"=w411:bool)  [unwired: 8 in]
          }
        }
        n164 = call <userlib>:"Log_basic.vi"("errin"=w396, "date?"=TRUE, "chaîne"=w401, "in"=w395) -> ("sortie d'erreur"=w397:errorcluster, "refnum en sortie"=w394:refnum<file>)  [unwired: 6 in]
        n165 = Compound Arithmetic op=AND ("Opérateur arithmétique")(w390) -> (w389:bool)
        n166 = Select ("Sélectionner")(t=OP500Z8_state_P."OCV" ("cas vrai"), s=w389, f=OP500Z8_state_P."Crash" ("Énum")) -> (s? t:f=w386:T7)
      }
      frame "OCV" {
        n167 = call <userlib>:"OUINONV2.vi"("errin"=w463, "image"="DCIR" ("IN")) -> ("error out"=w462:errorcluster)  [unwired: 8 in, 1 out]
        n168 = local read "VISA OUT"() -> (w467:T2)
        n169 = Unbundle By Name(w467) -> ("ITECH"=w466:refnum<visa-resource-name>)
        n170 = call "VerifPreDCIR_P.vi"("errin"=w462, "VISA resource name"=w466) -> ("errout"=w472:errorcluster, "Actual Voltage Level (V)"=w465:dbl, "V>10 ?"=w461:bool)  [unwired: 6 in, 1 out]
        n171 = local write "TOP"("Mesure de la tension à vide" ("TOP")) -> ()
        n172 = call <userlib>:"waitXms.vi"("attente (ms)"=u32 200, "errin"=w472) -> ("errout"=w468:errorcluster)  [unwired: 13 in]
        n173 = global read "VG_OCV70min_P.vi" "OCV70min"() -> (w476:dbl)
        n174 = global read "VG_OCV70max_P.vi" "OCV70max"() -> (w477:dbl)
        n175 = In Range and Coerce(upper limit=w477, x=w465, lower limit=w476) -> (In Range?=w479:bool)  [unwired: 1 out]
        n176 = global read "VG_OCV30max_P.vi" "OCV30max"() -> (w475:dbl)
        n177 = global read "VG_OCV30min_P.vi" "OCV30min"() -> (w474:dbl)
        n178 = In Range and Coerce(upper limit=w475, x=w465, lower limit=w474) -> (In Range?=w478:bool)  [unwired: 1 out]
        "IS30% ?" <- w478
        n179 = Or(x=w478, y=w479) -> (x .or. y?=w471:bool)
        n180 = case shown="True" w471 {
          tunnel: w486 -> [w508 w515]
          tunnel: [w508 w514] -> w485
          tunnel: w488 -> [w507 w513]
          tunnel: [w507 w512] -> w484
          tunnel: w465 -> [_ w511]
          tunnel: ["0" w510] -> w480
          frame False {
          }
          frame True {
            n181 = Number To Fractional String(number=w511, precision (6)=i16 2 ("précision (6)")) -> (F-format string=w510:string)  [unwired: 2 in]
            n182 = Concatenate Strings("OCV;" ("chaîne"), w510) -> (w517:string)
            n183 = call <userlib>:"Log_basic.vi"("errin"=w515, "date?"=TRUE, "chaîne"=w517, "in"=w513) -> ("sortie d'erreur"=w514:errorcluster, "refnum en sortie"=w512:refnum<file>)  [unwired: 6 in]
          }
        }
        n184 = global write "IS30%_P.vi" "VG IS30% ?"(w478) -> ()
        n185 = case shown="False" w471 {
          tunnel: w468 -> [w492 w505]
          tunnel: [w489 w505] -> w470
          tunnel: [w491 OP500Z8_state_P."CurrentTest" ("Énum")] -> w469
          tunnel: w461 -> [w490 _]
          frame False {
            n186 = case shown="False" w490 {
              tunnel: w492 -> [w499 w503]
              tunnel: [w496 OP500Z8_state_P."Crash" ("Énum")] -> w491
              tunnel: [w498 w503] -> w489
              frame False {
                # "V < 10 ? -> 0"
                n187 = call <userlib>:"OUINONV2.vi"("errin"=w499, "image"="Refaire" ("IN")) -> ("error out"=w498:errorcluster, "Booléen"=w495:bool)  [unwired: 8 in]
                n188 = One Button Dialog(message="Verifier que le bouton du tiroir est bien sur DCIR, et que les contacteur sont fermés") -> ()  [unwired: 1 in, 1 out]
                n189 = Select(t=OP500Z8_state_P."OCV" ("Énum"), s=w495, f=OP500Z8_state_P."Crash") -> (s? t:f=w496:T7)
              }
              frame True {
                # "Si il mesure une tension >10V"
                n190 = One Button Dialog(message="Le pack est ni à 30% ni à 70%") -> ()  [unwired: 1 in, 1 out]
              }
            }
          }
          frame True {
            # "Next si tout est ok"
          }
        }
        n191 = local read "Cluster"() -> (w482:T3)
        n192 = Bundle By Name(cluster=w482, "OCV"=w480) -> (w481:T3)
        n193 = local write "Cluster"(w481) -> ()
      }
      frame "CurrentTest" {
        w528 = FALSE ("Caption")
        w531 = -174.0 ("Consigne")
        w534 = -100.0 ("Consigne")
        w540 = -50.0 ("Consigne")
        w541 = 174.0 ("Consigne")
        w537 = 100.0 ("Consigne")
        w519 = 50.0 ("Consigne")
        # "same current direction ?"
        # "Idle Current + compare current value"
        n194 = property on="Courant BMS (A)" class="DigNum (strict)"(error in=w524, "Caption"=TRUE) -> (error out=w523:errorcluster)  [unwired: 1 in, 1 out]
        n195 = local read "VISA OUT"() -> (w584:T2)
        n196 = property on="Consigne ITECH (A)" class="DigNum (strict)"(error in=w523, "DtSktMode"=0.0 ("Consigne"), "Caption"=TRUE) -> (error out=w522:errorcluster)  [unwired: 1 in, 1 out]
        n197 = Unbundle By Name(w584) -> ("ITECH"=w582:refnum<visa-resource-name>)
        n198 = call "OP500Z8P_CurrentCompare.vi"("errin"=w522, "Consigne"=0.0, "ITECH VISA NAME"=w582) -> ("errout"=w521:errorcluster, "BDU Current (A)"=w581:dbl, "BMS Current (A)"=w568:string)  [unwired: 4 in, 2 out]
        n199 = call "FGV_Image.vi"("Énum"=FGV."SET", "IN"="CurrentMeas") -> ()  [unwired: 9 in, 1 out]
        n200 = property on="Consigne ITECH (A)" class="DigNum (strict)"(error in=w521, "DtSktMode"=w519) -> (error out=w520:errorcluster)  [unwired: 1 in, 1 out]
        n201 = In Range and Coerce(upper limit=0.5, x=w581, lower limit=0.0) -> (In Range?=w555:bool)  [unwired: 1 out]
        n202 = call "OP500Z8P_CurrentCompare.vi"("errin"=w520, "Consigne"=w519, "ITECH VISA NAME"=w582) -> ("errout"=w539:errorcluster, "Courant OK ?"=w578:bool, "BMS Current (A)"=w567:string)  [unwired: 4 in, 2 out]
        n203 = property on="Consigne ITECH (A)" class="DigNum (strict)"(error in=w539, "DtSktMode"=w537) -> (error out=w538:errorcluster)  [unwired: 1 in, 1 out]
        n204 = call "OP500Z8P_CurrentCompare.vi"("errin"=w538, "Consigne"=w537, "ITECH VISA NAME"=w582) -> ("errout"=w545:errorcluster, "Courant OK ?"=w577:bool, "BMS Current (A)"=w565:string)  [unwired: 4 in, 2 out]
        n205 = property on="Consigne ITECH (A)" class="DigNum (strict)"(error in=w545, "DtSktMode"=w541) -> (error out=w544:errorcluster)  [unwired: 1 in, 1 out]
        n206 = local write "TOP"("Je compare les valeurs du courant BMS et de l'alim" ("TOP")) -> ()
        n207 = call "OP500Z8P_CurrentCompare.vi"("errin"=w544, "Consigne"=w541, "ITECH VISA NAME"=w582) -> ("errout"=w543:errorcluster, "Courant OK ?"=w576:bool, "BMS Current (A)"=w563:string)  [unwired: 4 in, 2 out]
        n208 = property on="Consigne ITECH (A)" class="DigNum (strict)"(error in=w543, "DtSktMode"=w540) -> (error out=w542:errorcluster)  [unwired: 1 in, 1 out]
        n209 = call "OP500Z8P_CurrentCompare.vi"("errin"=w542, "Consigne"=w540, "ITECH VISA NAME"=w582) -> ("errout"=w536:errorcluster, "Courant OK ?"=w575:bool, "BMS Current (A)"=w561:string)  [unwired: 4 in, 2 out]
        n210 = property on="Consigne ITECH (A)" class="DigNum (strict)"(error in=w536, "DtSktMode"=w534) -> (error out=w535:errorcluster)  [unwired: 1 in, 1 out]
        n211 = call "OP500Z8P_CurrentCompare.vi"("errin"=w535, "Consigne"=w534, "ITECH VISA NAME"=w582) -> ("errout"=w533:errorcluster, "Courant OK ?"=w574:bool, "BMS Current (A)"=w559:string)  [unwired: 4 in, 2 out]
        n212 = property on="Consigne ITECH (A)" class="DigNum (strict)"(error in=w533, "DtSktMode"=w531) -> (error out=w532:errorcluster)  [unwired: 1 in, 1 out]
        n213 = call "OP500Z8P_CurrentCompare.vi"("errin"=w532, "Consigne"=w531, "ITECH VISA NAME"=w582) -> ("errout"=w546:errorcluster, "Courant OK ?"=w573:bool, "BMS Current (A)"=w557:string)  [unwired: 4 in, 2 out]
        n214 = Compound Arithmetic op=AND(w578, w577, w576, w575, w574, w573) -> (w553:bool)
        n215 = Select(t="OK" ("string"), s=w553, f="NOK") -> (s? t:f=w551:string)
        n216 = Concatenate Strings("IdleCurrent;" ("string"), w568, ";50?;" ("string"), w567, ";100?;" ("string"), w565, ";174?;" ("string"), w563, ";-50?;" ("string"), w561, ";-100?;" ("string"), w559, ";-174?;" ("string"), w557, ";CurrentDir;" ("string"), w551) -> (w571:string)
        n217 = call <userlib>:"Log_basic.vi"("errin"=w588, "date?"=TRUE, "chaîne"=w571, "in"=w590) -> ("sortie d'erreur"=w587:errorcluster, "refnum en sortie"=w586:refnum<file>)  [unwired: 6 in]
        n218 = And(x=w553, y=w555) -> (x .and. y?=w554:bool)
        n219 = property on="Consigne ITECH (A)" class="DigNum (strict)"(error in=w546, "Caption"=w528) -> (error out=w530:errorcluster)  [unwired: 1 in, 1 out]
        n220 = flat-sequence {
          tunnel: [w592] -> w556
          tunnel: w554 -> [w591]
          tunnel: w529 -> [_]
          frame #0 {
            n221 = Select(t=OP500Z8_state_P."GoDCIR" ("Énum"), s=w591, f=OP500Z8_state_P."Crash") -> (s? t:f=w592:T7)
          }
        }
        n222 = property on="Courant BMS (A)" class="DigNum (strict)"(error in=w530, "Caption"=w528) -> (error out=w529:errorcluster)  [unwired: 1 in, 1 out]
      }
      frame "GoDCIR" {
        # "Lancer la DCIR : fermature des contacteurs + control ITECH + Logging"
        n223 = local write "TOP"("Test DCIR" ("TOP")) -> ()
        n224 = local read "VISA OUT"() -> (w599:T2)
        n225 = Unbundle By Name(w599) -> ("ITECH"=w595:refnum<visa-resource-name>)
        n226 = local read "Cluster"() -> (w598:T3)
        n227 = Unbundle By Name(w598) -> ("SN"=w597:string)
        n228 = disable-structure shown="Enabled" {
          disable-tunnel: w607 -> [w626 w676]
          disable-tunnel: [w623 w683] -> w605
          disable-tunnel: [w622 w684] -> w603
          disable-tunnel: w595 -> [_ w682]
          disable-tunnel: w597 -> [_ w681]
          disable-tunnel: w595 -> [_ w680]
          frame Disabled {
            n229 = case shown="True" {
              selector: _ -> [w644 _]
              tunnel: [w644 w647] -> w617
              tunnel: w626 -> [w643 w646]
              tunnel: [w643 w645] -> w619
              frame False {
              }
              frame True {
                n230 = call <userlib>:"OUINONV2.vi"("errin"=w646, "image"="BMS") -> ("error out"=w645:errorcluster, "Booléen"=w647:bool)  [unwired: 8 in]
              }
            }
            n231 = case shown="True" w617 {
              selector: w617 -> [w632 _]
              tunnel: [w632 w635] -> w616
              tunnel: w619 -> [w631 w634]
              tunnel: [w631 w633] -> w618
              frame False {
              }
              frame True {
                n232 = call <userlib>:"OUINONV2.vi"("errin"=w634, "image"="PCANVIEW") -> ("error out"=w633:errorcluster, "Booléen"=w635:bool)  [unwired: 8 in]
              }
            }
            n233 = case shown="True" w616 {
              selector: w616 -> [w650 _]
              tunnel: [w650 w653] -> w621
              tunnel: w618 -> [w649 w652]
              tunnel: [w649 w651] -> w620
              frame False {
              }
              frame True {
                n234 = call <userlib>:"OUINONV2.vi"("errin"=w652, "image"="DCIRON") -> ("error out"=w651:errorcluster, "Booléen"=w653:bool)  [unwired: 8 in]
              }
            }
            n235 = case shown="True" w621 {
              selector: w621 -> [w638 _]
              tunnel: [w637 w641] -> w630
              tunnel: [w638 w640] -> w629
              tunnel: w620 -> [w637 w639]
              frame False {
              }
              frame True {
                n236 = call <userlib>:"OUINONV2.vi"("errin"=w639, "image"="Logging") -> ("error out"=w641:errorcluster, "Booléen"=w640:bool)  [unwired: 8 in]
              }
            }
            n237 = case shown="True" w629 {
              selector: w629 -> [w667 _]
              tunnel: w630 -> [w668 w672]
              tunnel: [w668 w670] -> w625
              tunnel: [w667 w669] -> w628
              frame False {
              }
              frame True {
                n238 = call <userlib>:"OUINONV2.vi"("errin"=w672, "image"="Minuteur") -> ("error out"=w670:errorcluster, "Booléen"=w669:bool)  [unwired: 8 in]
              }
            }
            n239 = case shown="True" w628 {
              selector: w628 -> [w662 _]
              tunnel: [w662 w665] -> w627
              tunnel: w625 -> [w661 w664]
              tunnel: [w661 w663] -> w624
              frame False {
              }
              frame True {
                n240 = call <userlib>:"OUINONV2.vi"("errin"=w664, "image"="Decharge") -> ("error out"=w663:errorcluster, "Booléen"=w665:bool)  [unwired: 8 in]
              }
            }
            n241 = case shown="True" w627 {
              selector: w627 -> [w656 _]
              tunnel: [w656 w659] -> w623
              tunnel: w624 -> [w655 w658]
              tunnel: [w655 w657] -> w622
              frame False {
              }
              frame True {
                n242 = call <userlib>:"OUINONV2.vi"("errin"=w658, "image"="StopLogging") -> ("error out"=w657:errorcluster, "Booléen"=w659:bool)  [unwired: 8 in]
              }
            }
          }
          frame Enabled {
            n243 = call <userlib>:"waitXms.vi"("attente (ms)"=u32 500, "errin"=w676) -> ("errout"=w675:errorcluster)  [unwired: 13 in]
            n244 = call "VerifPreDCIR_P.vi"("errin"=w675, "VISA resource name"=w680) -> ("errout"=w678:errorcluster, "V>10 ?"=w673:bool)  [unwired: 6 in, 2 out]
            n245 = call <userlib>:"waitXms.vi"("attente (ms)"=u32 300, "errin"=w678) -> ("errout"=w677:errorcluster)  [unwired: 13 in]
            n246 = case shown="True" w673 {
              selector: w673 -> [w687 _]
              tunnel: [w686 w693] -> w684
              tunnel: [w687 w692] -> w683
              tunnel: w682 -> [_ w690]
              tunnel: w681 -> [_ w689]
              tunnel: w677 -> [w686 w688]
              frame False {
                n247 = One Button Dialog(message="Vérifier le branchement de la com, \net que le bouton du tiroir est bien sur DCIR ") -> ()  [unwired: 1 in, 1 out]
              }
              frame True {
                n248 = property on="progression" class="Slide (strict)"(error in=w688, "Visible"=TRUE) -> (error out=w691:errorcluster)  [unwired: 1 in, 1 out]
                n249 = flat-sequence {
                  tunnel: w691 -> [_]
                  frame #0 {
                    n250 = call "FGV_Image.vi"("Énum"=FGV."SET", "IN"="DCIR-EnCours") -> ()  [unwired: 9 in, 1 out]
                  }
                }
                n251 = call "OP500Z8P_ReadFromPDU.vi"("errin"=w691, "SN"=w689, "VISA ITECH Name ?"=w690) -> ("errout"=w693:errorcluster, "BMS OK ?"=w692:bool)  [unwired: 6 in, 1 out]
              }
            }
          }
        }
        n252 = disable-structure shown="Enabled" {
          disable-tunnel: w603 -> [w700 w707]
          disable-tunnel: w605 -> [w699 w708]
          disable-tunnel: [w698 w708] -> w604
          disable-tunnel: [w697 w707] -> w602
          frame Disabled {
            n253 = case shown="True" w699 {
              selector: w699 -> [w702 _]
              tunnel: [w702 w705] -> w698
              tunnel: w700 -> [w701 w704]
              tunnel: [w701 w703] -> w697
              frame False {
              }
              frame True {
                n254 = call <userlib>:"OUINONV2.vi"("errin"=w704, "image"="Charge") -> ("error out"=w703:errorcluster, "Booléen"=w705:bool)  [unwired: 8 in]
              }
            }
          }
          frame Enabled {
          }
        }
        n255 = flat-sequence {
          tunnel: [w615] -> w606
          tunnel: w604 -> [w612]
          tunnel: w600 -> [_]
          frame #0 {
            n256 = Select(t=OP500Z8_state_P."DataDyn" ("Énum"), s=w612, f=OP500Z8_state_P."GoDCIR" ("cas faux")) -> (s? t:f=w615:T7)
          }
        }
        n257 = property on="progression" class="Slide (strict)"(error in=w602, "Visible"=FALSE, "Value"=0.0 ("progression")) -> (error out=w600:errorcluster)  [unwired: 1 in, 1 out]
      }
      frame "DataDyn" {
        # "Ce VI est en cours...............\nIl faut attendre 3 secondes, si le sub_vi CSV Reader n'a rien comme sortie\n--------------> on passe à l'etape LogErr"
        # "recuperation des donnees du fichier logging"
        n258 = local read "Cluster"() -> (w739:T3)
        n259 = local write "TOP"("Analyse de données" ("TOP")) -> ()
        n260 = Unbundle By Name(w739) -> ("SN"=w737:string)
        n261 = Concatenate Strings("\\\\forseepower.com\\fr\\040 Production\\FR7 - Poitiers\\06 Production\\05. Electronique\\Documents Control lib\\Archives\\ZEN_8\\Contrôle pack 48P\\Controle DCIR\\", w737, ".csv" ("chaîne")) -> (w724:string)
        n262 = global read "VG_DCIR+OUIouNON_P.vi" "VG_DCIR+ ?"() -> (w712:bool)
        n263 = String To Path(string=w724) -> (path=w728:path)
        n264 = call "OP500_NEW CSV READER_P.vi"("errin"=w727, "DCIR+ ?"=w712, "Choisir le fichier CSV"=w728) -> ("sortie d'erreur"=w722:errorcluster, "cluster"=w725:T9)  [unwired: 5 in]
        n265 = local read "Cluster"() -> (w711:T3)
        n266 = call "SubDataDyn_P.vi"("cluster"=w725, "Cluster en entrée"=w711) -> ("Chaîne"=w730:string, "cluster de sortie"=w710:T10)  [unwired: 8 in]
        n267 = call <userlib>:"Log_basic.vi"("errin"=w736, "date?"=TRUE, "chaîne"=w730, "in"=w734) -> ("sortie d'erreur"=w735:errorcluster, "refnum en sortie"=w733:refnum<file>)  [unwired: 6 in]
        n268 = Unbundle By Name(w710) -> ("VCell Max"=w720:string, "Vcell Min"=w719:string, "NTC Max"=w717:string, "NTC Min"=w718:string, "SOH"=w709:string)
        n269 = local write "Cluster"(w710) -> ()
        n270 = call "Stall Data Flow.vim"("value in"=w722, "milliseconds to wait"=u32 200) -> ("value out"=w721:errorcluster)  [unwired: 1 out]
        n271 = call "DataDynOK"("SOH"=w709, "NTC Min"=w718, "NTC Max"=w717, "Vcell Min"=w719, "VCell Max"=w720) -> ("DataDynOK ?"=w713:bool)  [unwired: 6 in]
        n272 = Select(t=OP500Z8_state_P."DTC" ("Next"), s=w713, f=OP500Z8_state_P."Crash" ("cas faux")) -> (s? t:f=w715:T7)
      }
      frame "DTC" {
        # "Voir s'il Y a des DTC"
        n273 = local write "TOP"("Analyse les DTC" ("TOP")) -> ()
        n274 = local read "Cluster"() -> (w752:T3)
        n275 = Unbundle By Name(w752) -> ("si DTC"=w741:string)
        n276 = Equal?(x="", y=w741) -> (x = y?=w743:bool)
        n277 = Select(t="NO DTC" ("chaîne"), s=w743, f=w741) -> (s? t:f=w740:string)
        n278 = call <userlib>:"waitXms.vi"("attente (ms)"=u32 100, "errin"=w750) -> ("errout"=w749:errorcluster)  [unwired: 13 in]
        n279 = Concatenate Strings("DTC;" ("chaîne"), w740) -> (w753:string)
        n280 = call <userlib>:"Log_basic.vi"("date?"=TRUE, "chaîne"=w753, "in"=w757) -> ("refnum en sortie"=w756:refnum<file>)  [unwired: 7 in, 1 out]
        n281 = Select(t=OP500Z8_state_P."DCIR" ("Énum"), s=w743, f=OP500Z8_state_P."Crash" ("cas faux")) -> (s? t:f=w746:T7)
      }
      frame "DCIR" {
        w767 = ";" ("chaîne")
        # "Recuperation de la valeur DCIR"
        n282 = local read "Cluster"() -> (w784:T3)
        n283 = global read "VG_DCIR+OUIouNON_P.vi" "VG_DCIR+ ?"() -> (w764:bool)
        n284 = Unbundle By Name(w784) -> ("DCIR"=w782:string, "DCIR +"=w763:string)
        n285 = local write "TOP"("Analyse de la resistance interne" ("TOP")) -> ()
        n286 = Select(t=w763, s=w764, f="NA") -> (s? t:f=w765:string)
        n287 = global read "VG_DCIRmin_P.vi" "DCIRmin"() -> (w761:dbl)
        n288 = Concatenate Strings("DCIR-" ("chaîne"), w767, w782, w767, "DCIR+" ("string"), w767, w765, w767) -> (w786:string)
        n289 = Increment(x=w761) -> (x+1=w760:dbl)
        n290 = call <userlib>:"Log_basic.vi"("errin"=w783, "date?"=TRUE, "chaîne"=w786, "in"=w788) -> ("sortie d'erreur"=w790:errorcluster, "refnum en sortie"=w789:refnum<file>)  [unwired: 6 in]
        n291 = Number To Decimal String(number=w760) -> (decimal integer string=w759:string)  [unwired: 1 in]
        n292 = global read "VG_DCIRmax_P.vi" "DCIRmax"() -> (w772:dbl)
        n293 = Select(t=w763, s=w764, f=w759) -> (s? t:f=w762:string)
        n294 = Fract/Exp String To Number(string=w782) -> (number=w781:dbl)  [unwired: 3 in, 1 out]
        n295 = call <userlib>:"waitXms.vi"("attente (ms)"=u32 100, "errin"=w776) -> ("errout"=w775:errorcluster)  [unwired: 13 in]
        n296 = Fract/Exp String To Number(string=w762) -> (number=w773:dbl)  [unwired: 3 in, 1 out]
        n297 = In Range and Coerce(upper limit=w772, x=w781, lower limit=w761) -> (In Range?=w771:bool)  [unwired: 1 out]
        n298 = In Range and Coerce(upper limit=w772, x=w773, lower limit=w761) -> (In Range?=w770:bool)  [unwired: 1 out]
        n299 = And(x=w771, y=w770) -> (x .and. y?=w769:bool)
        n300 = Select(t=OP500Z8_state_P."FinVol" ("Énum"), s=w769, f=OP500Z8_state_P."Crash" ("Énum")) -> (s? t:f=w778:T7)
      }
      frame "FinVol" {
        w792 = i16 2 ("precision (6)")
        # "Recuperation de la valeur DCIR"
        n301 = local read "VISA OUT"() -> (w807:T2)
        n302 = Unbundle By Name(w807) -> ("ITECH"=w795:refnum<visa-resource-name>)
        n303 = call "VerifPreDCIR_P.vi"("errin"=w796, "VISA resource name"=w795) -> ("errout"=w797:errorcluster, "Actual Voltage Level (V)"=w793:dbl)  [unwired: 6 in, 2 out]
        n304 = call "FGV_PDU_P.vi"("errin"=w797, "Énum"=FGV_Enum."SET", "IN"=FALSE) -> ("errout"=w811:errorcluster)  [unwired: 7 in, 1 out]
        n305 = call <userlib>:"waitXms.vi"("attente (ms)"=u32 1000, "errin"=w811) -> ("errout"=w808:errorcluster)  [unwired: 13 in]
        n306 = local write "TOP"("Je ferme les contacteurs et je mesure le tension l'absence de la tension" ("TOP")) -> ()
        n307 = call "VerifPreDCIR_P.vi"("errin"=w808, "VISA resource name"=w795) -> ("errout"=w802:errorcluster, "Actual Current Level (A)"=w799:dbl)  [unwired: 6 in, 2 out]
        n308 = Equal To 0?(x=w799) -> (x = 0?=w803:bool)
        n309 = case shown="False" w803 {
          selector: w803 -> [_ w834]
          tunnel: w802 -> [w832 w835]
          tunnel: [w825 w835] -> w801
          tunnel: w795 -> [w826 _]
          tunnel: [w823 w834] -> w800
          tunnel: w799 -> [_ w833]
          tunnel: [w822 w833] -> w798
          frame False {
            # "Si pas 0  --> on refait un test avant aller au CRASH"
            n310 = call "FGV_PDU_P.vi"("errin"=w832, "Énum"=FGV_Enum."SET", "IN"=FALSE) -> ("errout"=w829:errorcluster)  [unwired: 7 in, 1 out]
            n311 = call <userlib>:"waitXms.vi"("attente (ms)"=u32 2000, "errin"=w829) -> ("errout"=w827:errorcluster)  [unwired: 13 in]
            n312 = call "VerifPreDCIR_P.vi"("errin"=w827, "VISA resource name"=w826) -> ("errout"=w825:errorcluster, "Actual Current Level (A)"=w822:dbl, "Actual Voltage Level (V)"=w824:dbl)  [unwired: 6 in, 1 out]
            n313 = Equal To 0?(x=w824) -> (x = 0?=w823:bool)
          }
          frame True {
            # "Si 0V -> tres bien --> Next"
          }
        }
        n314 = Number To Fractional String(number=w793, precision (6)=w792) -> (F-format string=w794:string)  [unwired: 2 in]
        n315 = Number To Fractional String(number=w798, precision (6)=w792) -> (F-format string=w806:string)  [unwired: 2 in]
        n316 = Concatenate Strings("FinalOCV;" ("string"), w794, ";FinalVol;" ("string"), w806) -> (w804:string)
        n317 = call <userlib>:"Log_basic.vi"("errin"=w817, "date?"=TRUE, "chaîne"=w804, "in"=w819) -> ("sortie d'erreur"=w821:errorcluster, "refnum en sortie"=w820:refnum<file>)  [unwired: 6 in]
        n318 = Select(t=OP500Z8_state_P."Demontage" ("Énum"), s=w800, f=OP500Z8_state_P."Crash" ("Énum")) -> (s? t:f=w814:T7)
      }
      frame "BuildSys" {
        # "Recuperation de la valeur DCIR"
        n319 = local write "TOP"("J'ouvre les contacteurs et je mesure le tension l'absence de la tension" ("TOP")) -> ()
        n320 = call <userlib>:"Log_basic.vi"("errin"=w842, "date?"=TRUE, "in"=w844) -> ("sortie d'erreur"=w846:errorcluster, "refnum en sortie"=w845:refnum<file>)  [unwired: 7 in]
        n321 = Select(t=OP500Z8_state_P."Demontage" ("Énum"), s=FALSE, f=OP500Z8_state_P."Crash" ("Énum")) -> (s? t:f=w839:T7)
      }
      frame "Demontage" {
        w852 = OP500Z8_state_P."Next"  # Énum
        n322 = local write "TOP"("Demontage du pack" ("TOP")) -> ()
        n323 = call <userlib>:"OUINONV2.vi"("errin"=w854, "image"="Demontage" ("IN")) -> ("error out"=w848:errorcluster, "Booléen"=w847:bool)  [unwired: 8 in]
        n324 = Select ("Sélectionner")(t=w852, s=w847, f=OP500Z8_state_P."Demontage" ("cas faux")) -> (s? t:f=w849:T7)
      }
      frame "Crash" {
        w871 = path "\\\\forseepower.com\\fr/040 Production/FR7 - Poitiers/06 Production/05. Electronique/Documents Control lib/Archives/ZEN_8/Contrôle pack 48P/PV OP500" ("chemin de la cible (utiliser une boîte de dialogue)")
        # "C:\\Users\\ELHAJJ\\OneDrive - FORSEE POWER\\Bureau\\PV ZEN8 TEST"
        # "On genère le PV et on ferme le programme"
        n325 = call "FGV_PDU_P.vi"("errin"=w862, "Énum"=FGV_Enum."SET", "IN"=FALSE) -> ("errout"=w861:errorcluster)  [unwired: 7 in, 1 out]
        n326 = Close File(refnum=w883, error in=w882) -> (path=w873:path, error out=w876:errorcluster)
        n327 = call <userlib>:"waitXms.vi"("attente (ms)"=u32 300, "errin"=w876) -> ("errout"=w874:errorcluster)  [unwired: 13 in]
        n328 = Read from Text File(file (use dialog)=w873, error in=w874) -> (error out=w870:errorcluster)  [unwired: 2 in, 3 out]
        n329 = call "Stall Data Flow.vim"("value in"=w861, "milliseconds to wait"=u32 1000) -> ("value out"=w860:errorcluster)  [unwired: 1 out]
        n330 = local read "VISA OUT"() -> (w866:T2)
        n331 = Unbundle By Name(w866) -> ("TENMA"=w865:refnum<visa-resource-name>)
        n332 = call "FGV_Image.vi"("Énum"=FGV."SET", "IN"="Crash") -> ()  [unwired: 9 in, 1 out]
        n333 = call "TENMA_Conf_On_P.vi"("errin"=w860, "Tenma On?"=FALSE, "Visa in tenma"=w865) -> ("sortie d'erreur"=w863:errorcluster)  [unwired: 7 in, 1 out]
        n334 = Copy ("Copier")(8:w870, 10:w871, 11:w873) -> (0:w875:errorcluster)  [unwired: 2 in, 2 out]
        n335 = call "PvgeneratorOP500P.vi"("errin"=w875, "network"=w871, "path in"=w873) -> ("sortie d'erreur"=w879:errorcluster, "network out"=w878:path)  [unwired: 5 in, 2 out]
        n336 = flat-sequence {
          tunnel: [w886] -> w884
          tunnel: w872 -> [_]
          tunnel: [OP500Z8_state_P."Null"] -> w867
          frame #0 {
            w886 = TRUE
            n337 = local write "STOP"(w886) -> ()
          }
        }
        n338 = call <userlib>:"POP_GOOGLE.vi"("error in"=w879, "chemin"=w878) -> ("error out"=w872:errorcluster)  [unwired: 8 in, 1 out]
      }
      frame "Next" {
        w902 = path "\\\\forseepower.com\\fr/040 Production/FR7 - Poitiers/06 Production/05. Electronique/Documents Control lib/Archives/ZEN_8/Contrôle pack 48P/PV OP500" ("chemin de la cible (utiliser une boîte de dialogue)")
        w912 = OP500Z8_state_P."EXIT"  # Énum
        w913 = OP500Z8_state_P."Scan"  # Énum
        n339 = call <userlib>:"OUINONV2.vi"("errin"=w898, "image"="PassOrFail" ("IN")) -> ("error out"=w897:errorcluster, "Booléen"=w896:bool)  [unwired: 8 in]
        n340 = Close File(refnum=w915, error in=w914) -> (path=w905:path, error out=w911:errorcluster)
        n341 = case shown="True" w896 {
          selector: w896 -> [w934 _]
          tunnel: w897 -> [w935 w938]
          tunnel: [w934 w937] -> w894
          tunnel: [w935 w936] -> w893
          frame False {
          }
          frame True {
            n342 = call <userlib>:"OUINONV2.vi"("errin"=w938, "image"="EttJaune" ("IN")) -> ("error out"=w936:errorcluster, "Booléen"=w937:bool)  [unwired: 8 in]
          }
        }
        n343 = call <userlib>:"waitXms.vi"("attente (ms)"=u32 300, "errin"=w911) -> ("errout"=w907:errorcluster)  [unwired: 13 in]
        n344 = Read from Text File(file (use dialog)=w905, error in=w907) -> (error out=w901:errorcluster)  [unwired: 2 in, 3 out]
        n345 = case shown="True" w894 {
          selector: w894 -> [w929 _]
          tunnel: w893 -> [w928 w932]
          tunnel: [w929 w931] -> w895
          tunnel: [w928 w930] -> w892
          frame False {
          }
          frame True {
            n346 = call <userlib>:"OUINONV2.vi"("errin"=w932, "image"="EttBleu" ("IN")) -> ("error out"=w930:errorcluster, "Booléen"=w931:bool)  [unwired: 8 in]
          }
        }
        n347 = case shown="True" w895 {
          selector: w895 -> [w923 _]
          tunnel: w892 -> [w922 w926]
          tunnel: [w923 w925] -> w889
          tunnel: [w922 w924] -> w891
          frame False {
          }
          frame True {
            n348 = call <userlib>:"OUINONV2.vi"("errin"=w926, "image"="eProd" ("IN")) -> ("error out"=w924:errorcluster, "Booléen"=w925:bool)  [unwired: 8 in]
          }
        }
        n349 = Copy ("Copier")(8:w901, 10:w902, 11:w905) -> (0:w906:errorcluster)  [unwired: 2 in, 2 out]
        n350 = call "PvgeneratorOP500P.vi"("errin"=w906, "network"=w902, "path in"=w905) -> ("sortie d'erreur"=w909:errorcluster, "network out"=w908:path)  [unwired: 5 in, 2 out]
        n351 = case shown="True" w889 {
          selector: w889 -> [w917 _]
          tunnel: w891 -> [w916 w920]
          tunnel: [w917 w919] -> w888
          tunnel: [w916 w918] -> w890
          frame False {
          }
          frame True {
            n352 = call <userlib>:"OUINONV2.vi"("errin"=w920, "image"="ProdOF" ("IN")) -> ("error out"=w918:errorcluster, "Booléen"=w919:bool)  [unwired: 8 in]
          }
        }
        n353 = call <userlib>:"POP_GOOGLE.vi"("error in"=w909, "chemin"=w908) -> ("error out"=w903:errorcluster)  [unwired: 8 in, 1 out]
        n354 = case shown="True" w888 {
          selector: w888 -> [w941 _]
          tunnel: [w940 w944] -> w887
          tunnel: w890 -> [w940 w942]
          tunnel: [w941 w943] -> w900
          frame False {
          }
          frame True {
            n355 = call <userlib>:"OUINONV2.vi"("errin"=w942, "image"="Next" ("IN")) -> ("error out"=w944:errorcluster, "Booléen"=w943:bool)  [unwired: 8 in]
          }
        }
        n356 = Select(t=w913, s=w900, f=w912) -> (s? t:f=w904:T7)
      }
      frame "EXIT" {
        # "Eteindre le banc avant de quitter labview"
        n357 = call <userlib>:"OUINONV2.vi"("errin"=w951, "image"="TurnOff" ("IN")) -> ("error out"=w950:errorcluster, "Booléen"=w949:bool)  [unwired: 8 in]
        n358 = Select(t=OP500Z8_state_P."EXIT" ("cas vrai"), s=w949, f=OP500Z8_state_P."Null" ("Énum")) -> (s? t:f=w947:T7)
        n359 = flat-sequence {
          tunnel: w950 -> [_]
          frame #0 {
            n360 = Quit LabVIEW(quit? (T)=TRUE ("quitter ? (V)")) -> ()
          }
        }
      }
      frame "LogErr" {
        # "En cours.................................................................................................."
        # "au cas ou le fichier de log n'existe pas ou il contient pas le test DCIR"
        n361 = call <userlib>:"OUINONV2.vi"("errin"=w957, "image"="LogErr") -> ("error out"=w958:errorcluster, "Booléen"=w956:bool)  [unwired: 8 in]
        n362 = Select(t=OP500Z8_state_P."GoDCIR" ("cas vrai"), s=w956, f=OP500Z8_state_P."Crash" ("Énum")) -> (s? t:f=w959:T7)
      }
    }
    n363 = Wait (ms)(milliseconds to wait=u32 200 ("attente (ms)")) -> ()  [unwired: 1 out]
    n364 = case shown="True" w44 {
      selector: w44 -> [_ w51]
      frame False {
      }
      frame True {
        n365 = local write "STOP"(w51) -> ()
      }
    }
  }
  n366 = while {
    tunnel: errorcluster {"status"=FALSE, "code"=0, "source"=""} ("error out") -> [w970]
    tunnel: [w963] -> _
    stop <- w964 stop-if-true
    # "ici tu met l'image à jour si besoin"
    n367 = Wait (ms)(milliseconds to wait=u32 200 ("attente (ms)")) -> ()  [unwired: 1 out]
    n368 = call "FGV_Image.vi"("Énum"=FGV."GET") -> ("OUT"=w966:string)  [unwired: 10 in]
    n369 = Not Equal?(x=w966, y="") -> (x != y?=w967:bool)
    n370 = case shown="False" w967 {
      tunnel: [w972 w976] -> w963
      tunnel: w970 -> [w972 w975]
      tunnel: w966 -> [_ w974]
      frame False {
      }
      frame True {
        n371 = call <vilib>:"Application Directory.vi"() -> ("Application Directory"=w979:path)
        n372 = Path To String(path=w979) -> (string=w980:string)
        n373 = Concatenate Strings(w980, "\\Image\\" ("chaîne"), w974, ".jpg" ("chaîne")) -> (w978:string)
        n374 = String To Path(string=w978) -> (path=w977:path)
        n375 = call <vilib>:"Read JPEG File.vi"("error in (no error)"=w975, "path to JPEG file"=w977) -> ("error out"=w976:errorcluster, "image data"=w983:T11)  [unwired: 7 in, 1 out]
        n376 = call <vilib>:"Draw Flattened Pixmap.vi"("image data"=w983) -> ("new picture"=w973:picture)  [unwired: 8 in]
        n377 = local write "DRAW"(w973) -> ()
      }
    }
    n378 = global read "VG_progressBar_P.vi" "progression"() -> (→"progression":dbl)
    n379 = global read "VG_Barre_Progression_ISO_P.vi" "VG_Barre_Progression"() -> (→"Barre de progression ISO":dbl)
    n380 = global read "VG_Ibms.vi" "VG_Ibms"() -> (→"Courant BMS (A)":dbl)
    n381 = local read "STOP"() -> (w964:bool)
  }
  n382 = while {
    i -> [w987]
    stop <- w984 stop-if-true
    # "FGV pour led Alarm"
    n383 = local read "STOP"() -> (w984:bool)
    n384 = Wait (ms)(milliseconds to wait=u32 500) -> ()  [unwired: 1 out]
    n385 = call "OP500Z8_FGV_Alarm_P.vi"("Énum"=FGV_Enum."GET") -> ("OUT"=w985:bool)  [unwired: 9 in, 1 out]
    n386 = case shown="True" w985 {
      tunnel: w987 -> [_ w989]
      frame False {
      }
      frame True {
        n387 = Quotient & Remainder(x=w989, y=2) -> (x-y*floor(x/y)=w992:i32)  [unwired: 1 out]
        n388 = Not Equal?(x=0, y=w992) -> (x != y?=→"Boolean":bool)
      }
    }
  }
  n389 = call <userlib>:"PEAK_Init_plus.vi"("Channel"=Channel."PCAN_USBBUS1", "BTR0BTR1"=BaudrateEenum."CAN_BAUD_500K") -> ("errout"=w4:errorcluster, "Channel out"=w3:T4)  [unwired: 8 in]
  n390 = while {
    tunnel: w4 -> [w995]
    tunnel: w3 -> [w1000]
    tunnel: [w997] -> w2
    tunnel: [w999] -> w1
    stop <- w998 stop-if-true
    # "Trame PC->PDU : fermeture des contacteurs"
    n391 = call "FGV_PDU_P.vi"("Énum"=FGV_Enum."GET") -> ("OUT"=w1001:bool)  [unwired: 9 in, 1 out]
    n392 = case shown="No Error" w995 {
      tunnel: w1001 -> [w1007 _]
      tunnel: w995 -> [w1006 w1017]
      tunnel: w1000 -> [w1005 w1016]
      tunnel: [w1004 w1016] -> w999
      tunnel: [w1003 w1017] -> w997
      frame No Error {
        n393 = case shown="True" w1007 {
          tunnel: w1006 -> [w1009 w1015]
          tunnel: w1005 -> [w1008 w1013]
          tunnel: [w1009 w1014] -> w1003
          tunnel: [w1008 w1013] -> w1004
          frame False {
          }
          frame True {
            n394 = call <userlib>:"PEAK_Can_Write.vi"("CAN Handle"=w1013, "MSG type"=enum8{"STD", "RTR", "XTD", "XTD RTR", "STATUS"}."XTD", "errin"=w1015, "CAN Data"=u8[] [1, 0, 0, 0, 0, 0, 0, 0], "Identifier"=u32 419398788) -> ("errout"=w1014:errorcluster)  [unwired: 6 in]
          }
        }
      }
      frame Error {
      }
    }
    n395 = local read "STOP"() -> (w996:bool)
    n396 = Or(x=w997, y=w996) -> (x .or. y?=w998:bool)
    n397 = Wait (ms) ("Attendre (ms)")(milliseconds to wait=u32 150 ("attente (ms)")) -> ()  [unwired: 1 out]
  }
  n398 = while {
    tunnel: [w1023] -> _
    stop <- w1019 stop-if-true
    # "FGV pour lire le courant de la tenma"
    n399 = local read "VISA OUT"() -> (w1022:T2)
    n400 = local read "STOP"() -> (w1019:bool)
    n401 = Unbundle By Name(w1022) -> ("TENMA"=w1021:refnum<visa-resource-name>)
    n402 = call "OP500Z8P_TenmaReadCurr.vi"("Visa in tenma"=w1021) -> ("sortie d'erreur"=w1023:errorcluster, "I tenma (A)"=w1020:dbl, "cont fermés ?"=→"Contacteur Status":bool)  [unwired: 6 in, 2 out]
    n403 = Wait (ms)(milliseconds to wait=u32 600) -> ()  [unwired: 1 out]
    n404 = call "FGV_TENMAread.vi"("Énum"=FGV_Enum."SET", "Numeric input"=w1020) -> ()  [unwired: 8 in, 2 out]
  }
  n405 = call <userlib>:"CAN Uninitialize.vi"("error in (no error)"=w2, "Channel"=w1) -> ("error out"=w15:errorcluster)  [unwired: 7 in, 2 out]
  n406 = Merge Errors(w36, w35, w15) -> (→"errout":errorcluster)
  "STOP" <- w33
